vi "单参数加标流程.vi"(10 "流程类型":T4, 11 "Slave ID":T6=enum."氨氮") -> ()   [LabVIEW 2016, in "质控单元V4.lvlib"]
panel:
  in  "平行样测试数据":T1={"时间"=timestamp(0 s since 1904-01-01), "参数"="", "数据类型"="N", "第一次水样浓度值"=0.0, "第二次水样测试时间"=timestamp(0 s since 1904-01-01), "第二次水样浓度值"=0.0}
  in  "集成干预测试数据":T2={"时间"=timestamp(0 s since 1904-01-01), "参数"="", "数据类型"="N", "集成干预测试浓度值"=0.0, "集成干预前测试时间"=timestamp(0 s since 1904-01-01), "集成干预前测试浓度值"=0.0}
  out "平行样启动时间":timestamp
  out "加标模块润洗流程控制":T3=enum."启动水样润洗流程"
  in  "获取加标回收测试数据计数":u16
  in  "获取水样测试数据计数":u16
  in  "写入加标体积重试次数":u16
  in  "加标模块加标润洗启动计数":u16
  out "加标回收启动时间":timestamp
  out "水样测试启动时间":timestamp
  out "Next State":string
  in  "仪器加标回收启动计数":u16
  in  "仪器水样测试启动计数":u16
  in  "加标模块排液启动计数":u16
  in  "加标模块加标启动计数":u16
  in  "加标模块进样启动计数":u16
  in  "加标模块水样润洗启动计数":u16
  in  "采配水启动次数计数":u16
  in  "加标回收测试时间":timestamp
  in  "水样测试时间":timestamp
  in  "质控数据":T5
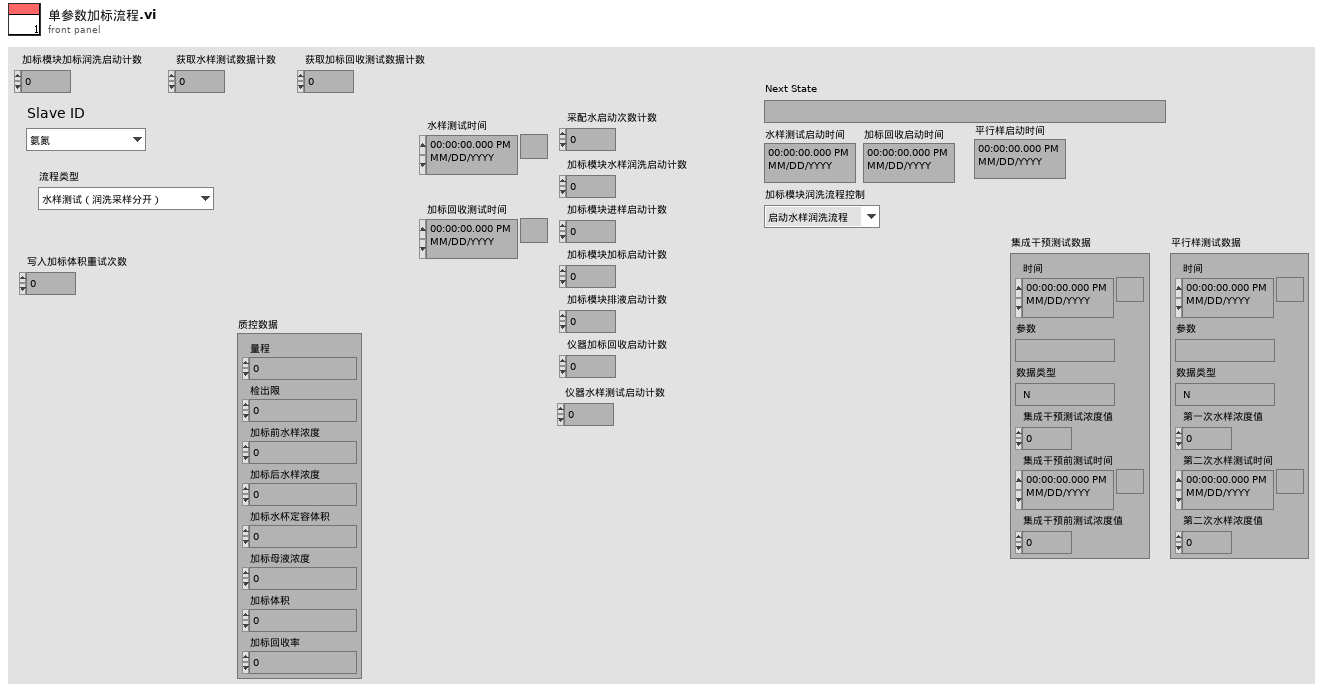
[diagram p1: front panel]
types:
  T1 = typedef "平行样测试数据字段定义.ctl" = cluster{"时间":timestamp, "参数":string, "数据类型":string, "第一次水样浓度值":dbl, "第二次水样测试时间":timestamp, "第二次水样浓度值":dbl}
  T2 = typedef "集成干预字段定义.ctl" = cluster{"时间":timestamp, "参数":string, "数据类型":string, "集成干预测试浓度值":dbl, "集成干预前测试时间":timestamp, "集成干预前测试浓度值":dbl}
  T3 = typedef "质控单元V4.lvlib/质控流程控制.ctl" = enum16{"待机", "启动进样流程", "启动加标流程", "启动排液流程", "启动水样润洗流程", "启动加标润洗流程", "停止流程"}
  T4 = typedef "质控单元V4.lvlib/测试子流程.ctl" = enum16{"水样测试（润洗采样分开）", "水样测试（润洗采样合并）", "水样测试（不启动采配水）", "加标回收（润洗采样分开）", "加标回收（润洗采样合并）", "加标回收（不启动采配水）", "集成干预测试", "平行样测试", "平行样测试（不启动采配水）", "水样测试（不含采样杯）", "平行样测试（不含采样杯）", "集成干预测试（不含采样杯）"}
  T5 = cluster{"量程":dbl, "检出限":dbl, "加标前水样浓度":dbl, "加标后水样浓度":dbl, "加标水杯定容体积":dbl, "加标母液浓度":dbl, "加标体积":dbl, "加标回收率":dbl}
  T6 = typedef "质控单元V4.lvlib/质控slave id.ctl" = enum16{"null", "氨氮", "总磷", "总氮", "CODMn", "CODCr"}
  T7 = cluster{"氨氮":bool, "总磷":bool, "总氮":bool, "CODMn":bool, "CODCr":bool}
  T8 = cluster{"时间":timestamp, "参数":string, "数据类型":string, "加标回收率":sgl, "加标前水样测试时间":timestamp, "加标前水样浓度值":sgl, "加标后水样浓度值":sgl, "加标母液浓度值":sgl, "加标体积":sgl, "加标水杯定容体积":sgl}
  T9 = enum16{"待机", "水样测试（全流程）", "停止", "加标回收", "水样测试（简易流程）"}
  T10 = enum16{"待机", "润洗", "采样", "沉淀", "配水", "反冲洗", "储水", "结束"}
  T11 = typedef "质控单元V4.lvlib/采配水通用流程.ctl" = enum16{"待机", "润洗", "采样", "沉淀", "配水", "反冲洗", "结束"}
  T12 = typedef "质控单元V4.lvlib/质控组合命令区.ctl" = enum16{"停止", "进水样", "排废液", "进空气（搅拌）", "定量（反转定量）"}
  T13 = enum16{"待机", "润洗", "进样", "定量", "加标", "等待取样", "排液", "异常停机"}
  T14 = enum16{"空闲", "水样测试", "标样核查", "零点核查", "跨度核查", "空白测试", "平行样测试", "加标回收", "空白校准", "标样校准", "初始化（清洗）"}
  T15 = cluster{"时间":timestamp, "参数":string, "数据类型":string, "第一次水样浓度值":dbl, "第二次水样测试时间":timestamp, "第二次水样浓度值":dbl}
  T16 = cluster{"水样数据时间":timestamp, "水样实测值":sgl, "水样数据标识":string}
  T17 = cluster{"加标回收数据时间":timestamp, "加标回收实测值":sgl, "加标回收数据标识":string}
  T18 = typedef "质控单元V4.lvlib/质控仪器状态.ctl" = cluster{"运行状态":enum16{"待机", "润洗", "进样", "定量", "加标", "等待取样", "排液", "异常停机"}, "液位状态":enum16{"无感应", "有感应"}, "告警状态":enum16{"无告警", "液位故障告警", "注射泵异常"}, "当前步骤数":u16, "当前步骤剩余时间":u16, "当前步骤具体操作":enum16{"加标", "进样", "排液", "搅拌", "定量"}, "当前流程":enum16{"待机", "进样流程", "加标流程", "排液流程", "水样润洗流程", "加标润洗流程"}}
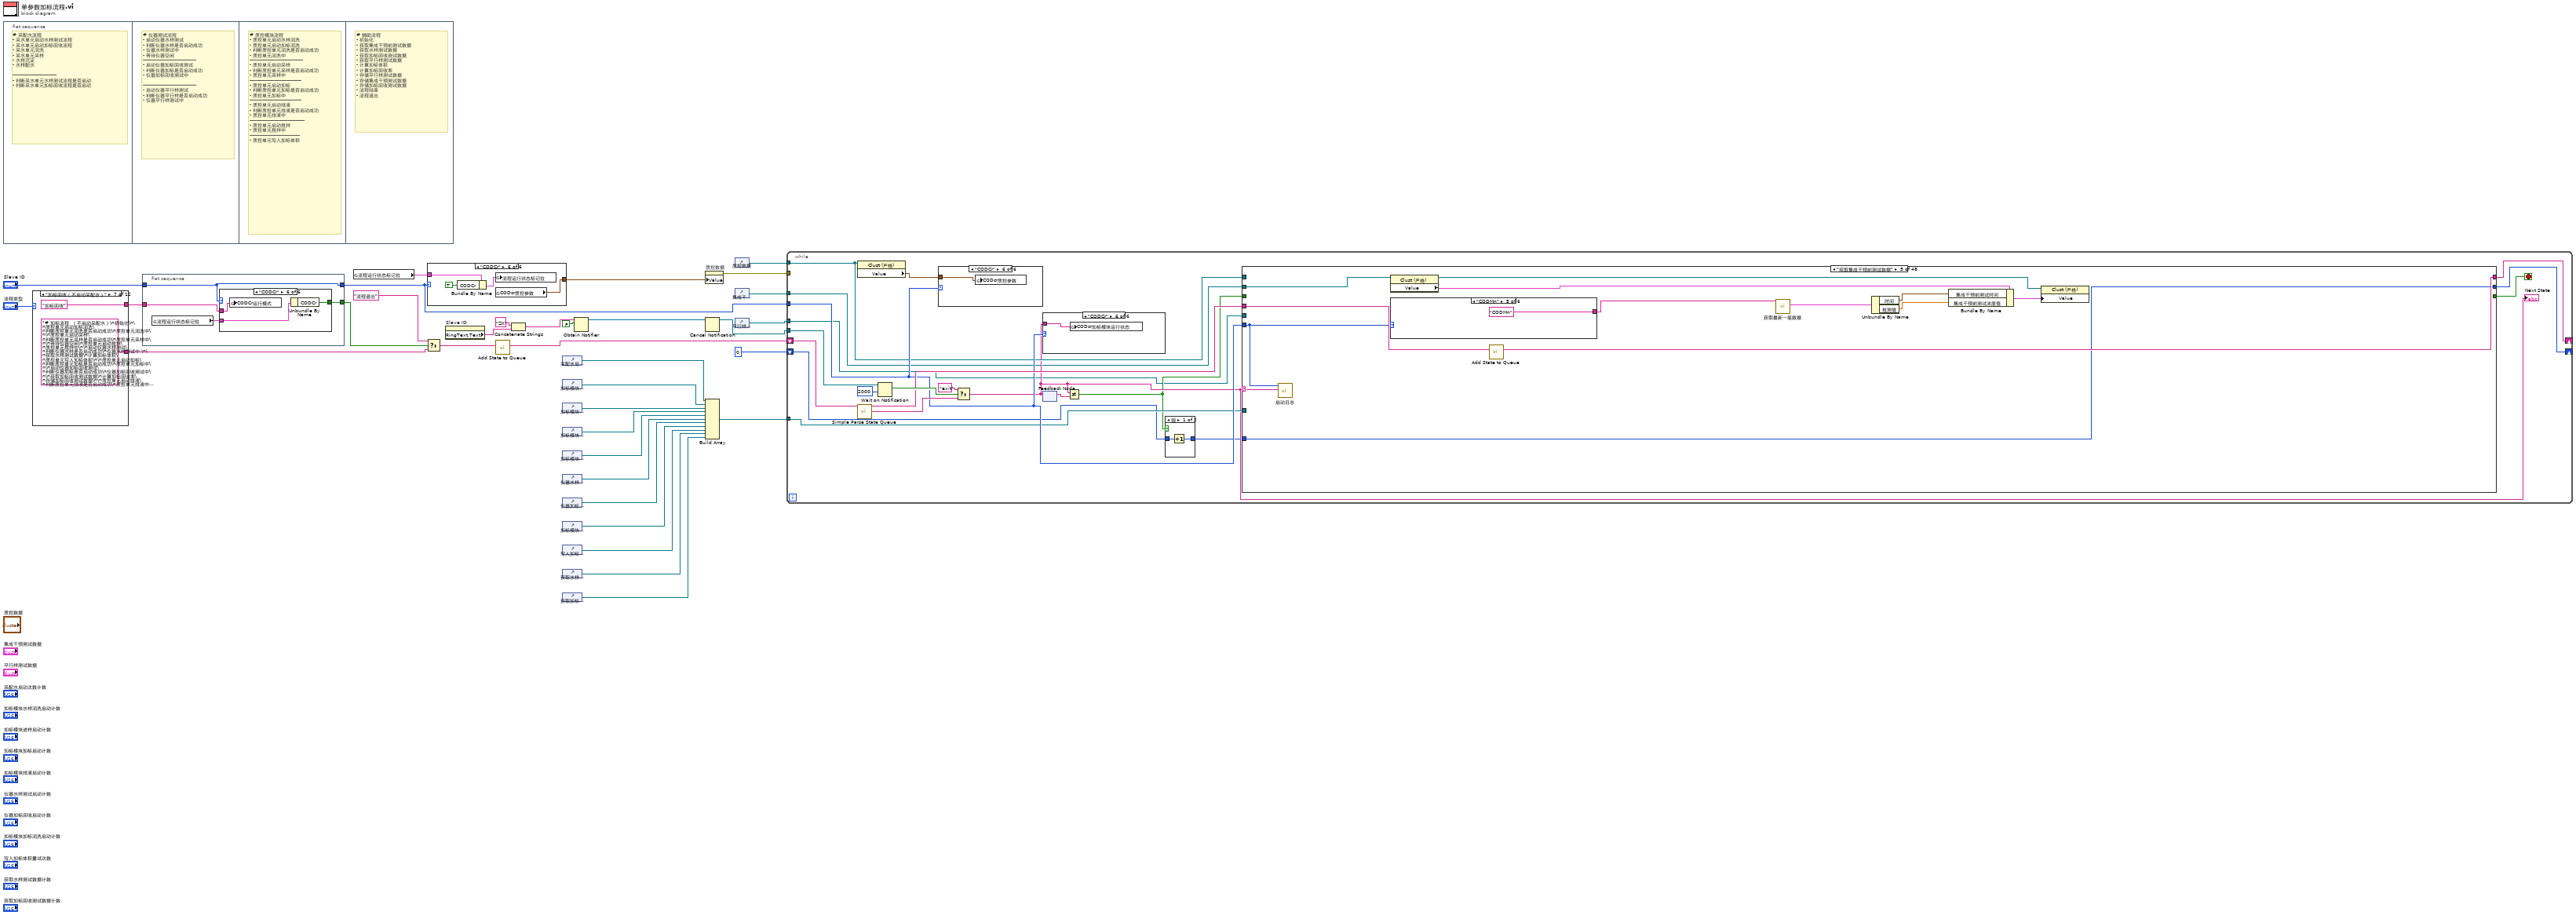
[diagram p0: block diagram]
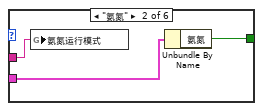
[diagram p3: hidden frame]
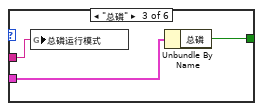
[diagram p4: hidden frame]
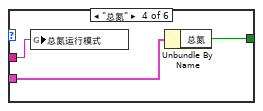
[diagram p5: hidden frame]
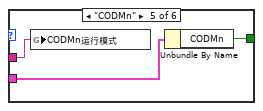
[diagram p6: hidden frame]
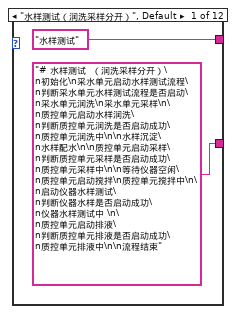
[diagram p7: hidden frame]
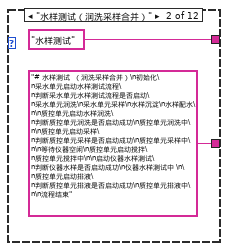
[diagram p8: hidden frame]
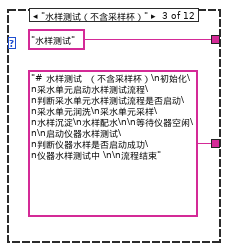
[diagram p9: hidden frame]
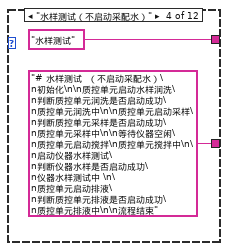
[diagram p10: hidden frame]
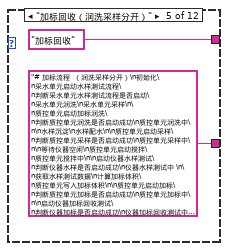
[diagram p11: hidden frame]
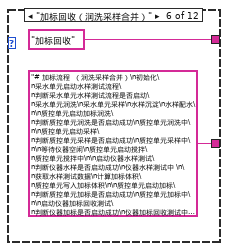
[diagram p12: hidden frame]
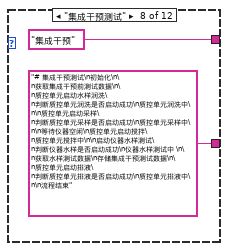
[diagram p13: hidden frame]
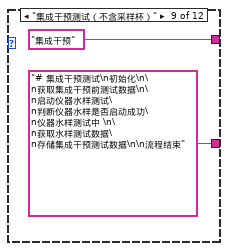
[diagram p14: hidden frame]
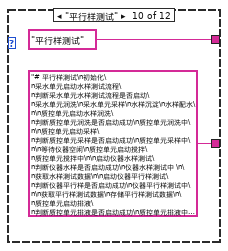
[diagram p15: hidden frame]
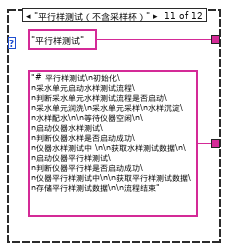
[diagram p16: hidden frame]
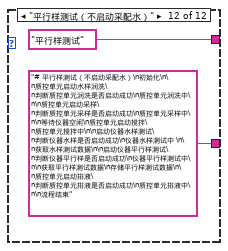
[diagram p17: hidden frame]
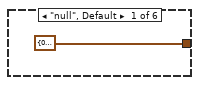
[diagram p18: hidden frame]
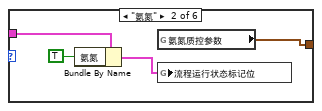
[diagram p19: hidden frame]
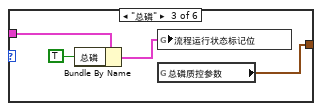
[diagram p20: hidden frame]
diagram:
  n1 = flat-sequence {
    frame #0 {
      # "# 采配水流程\n- 采水单元启动水样测试流程\n- 采水单元启动加标回收流程\n- 采水单元润洗\n- 采水单元采样 \n- 水样沉淀\n- 水样配水\n\n----------------------------\n- 判断采水单元水样测试流程是否启动\n- 判断采水单元加标回收流程是否启动"
    }
    frame #1 {
      # "# 仪器测试流程\n- 启动仪器水样测试\n- 判断仪器水样是否启动成功\n- 仪器水样测试中\n- 等待仪器空闲\n----------------------------------\n- 启动仪器加标回收测试\n- 判断仪器加标是否启动成功\n- 仪器加标回收测试中\n\n----------------------------------\n- 启动仪器平行样测试\n- 判断仪器平行样是否启动成功\n- 仪器平行样测试中"
    }
    frame #2 {
      # "# 质控模块流程\n- 质控单元启动水样润洗\n- 质控单元启动加标润洗\n- 判断质控单元润洗是否启动成功\n- 质控单元润洗中\n----------------------------------\n- 质控单元启动采样\n- 判断质控单元采样是否启动成功\n- 质控单元采样中\n---------------------------------\n- 质控单元启动加标\n- 判断质控单元加标是否启动成功\n- 质控单元加标中\n---------------------------------\n- 质控单元启动排液\n- 判断质控单元排液是否启动成功\n- 质控单元排液中\n-----------------------------------\n- 质控单元启动搅拌\n- 质控单元搅拌中\n--------------------------------\n- 质控单元写入加标体积"
    }
    frame #3 {
      # "# 辅助流程\n- 初始化\n- 获取集成干预前测试数据\n- 获取水样测试数据\n- 获取加标回收测试数据\n- 获取平行样测试数据\n- 计算加标体积\n- 计算加标回收率\n- 存储平行样测试数据\n- 存储集成干预测试数据\n- 存储加标回收测试数据 \n- 流程结束\n- 流程退出"
    }
  }
  n2 = case shown="\"加标回收（不启动采配水）\"" "流程类型" {
    tunnel: ["# 水样测试  （润洗采样分开）\n初始化\n采水单元启动水样测试流程\n判断采水单元水样测试流程是否启动\n采水单元润洗\n采水单元采样\n\n质控单元启动水样润洗\n判断质控单元润洗是否启动成功\n质控单元润洗中\n\n水样沉淀\n水样配水\n\n质控单元启动采样\n判断质控单元采样是否启动成功\n质控单元采样中\n\n等待仪器空闲\n质控单元启动搅拌\n质控单元搅拌中\n\n启动仪器水样测试\n判断仪器水样是否启动成功\n仪器水样测试中 \n\n质控单元启动排液\n判断质控单元排液是否启动成功\n质控单元排液中\n\n流程结束" ("State(s) In (\"\")") "# 水样测试  （润洗采样合并）\n初始化\n采水单元启动水样测试流程\n判断采水单元水样测试流程是否启动\n采水单元润洗\n采水单元采样\n水样沉淀\n水样配水\n\n质控单元启动水样润洗\n判断质控单元润洗是否启动成功\n质控单元润洗中\n\n质控单元启动采样\n判断质控单元采样是否启动成功\n质控单元采样中\n\n等待仪器空闲\n质控单元启动搅拌\n质控单元搅拌中\n\n启动仪器水样测试\n判断仪器水样是否启动成功\n仪器水样测试中 \n\n质控单元启动排液\n判断质控单元排液是否启动成功\n质控单元排液中\n\n流程结束" ("State(s) In (\"\")") "# 水样测试  （不含采样杯）\n初始化\n采水单元启动水样测试流程\n判断采水单元水样测试流程是否启动\n采水单元润洗\n采水单元采样\n水样沉淀\n水样配水\n\n等待仪器空闲\n\n启动仪器水样测试\n判断仪器水样是否启动成功\n仪器水样测试中 \n\n流程结束" ("State(s) In (\"\")") "# 水样测试  （不启动采配水）\n初始化\n\n质控单元启动水样润洗\n判断质控单元润洗是否启动成功\n质控单元润洗中\n\n质控单元启动采样\n判断质控单元采样是否启动成功\n质控单元采样中\n\n等待仪器空闲\n质控单元启动搅拌\n质控单元搅拌中\n\n启动仪器水样测试\n判断仪器水样是否启动成功\n仪器水样测试中 \n\n质控单元启动排液\n判断质控单元排液是否启动成功\n质控单元排液中\n\n流程结束" ("State(s) In (\"\")") "# 加标流程  （润洗采样分开）\n初始化\n采水单元启动水样测试流程\n判断采水单元水样测试流程是否启动\n采水单元润洗\n采水单元采样\n\n质控单元启动加标润洗\n判断质控单元润洗是否启动成功\n质控单元润洗中\n\n水样沉淀\n水样配水\n\n质控单元启动采样\n判断质控单元采样是否启动成功\n质控单元采样中\n\n等待仪器空闲\n质控单元启动搅拌\n质控单元搅拌中\n\n启动仪器水样测试\n判断仪器水样是否启动成功\n仪器水样测试中 \n\n获取水样测试数据\n计算加标体积\n质控单元写入加标体积\n\n质控单元启动加标\n判断质控单元加标是否启动成功\n质控单元加标中\n\n启动仪器加标回收测试\n判断仪器加标是否启动成功\n仪器加标回收测试中\n\n获取加标回收测试数据\n计算加标回收率\n存储加标回收测试数据\n\n质控单元启动排液\n判断质控单元排液是否启动成功\n质控单元排液中\n\n流程结束" ("State(s) In (\"\")") "# 加标流程  （润洗采样合并）\n初始化\n采水单元启动水样测试流程\n判断采水单元水样测试流程是否启动\n采水单元润洗\n采水单元采样\n水样沉淀\n水样配水\n\n质控单元启动加标润洗\n判断质控单元润洗是否启动成功\n质控单元润洗中\n\n质控单元启动采样\n判断质控单元采样是否启动成功\n质控单元采样中\n\n等待仪器空闲\n质控单元启动搅拌\n质控单元搅拌中\n\n启动仪器水样测试\n判断仪器水样是否启动成功\n仪器水样测试中 \n\n获取水样测试数据\n计算加标体积\n质控单元写入加标体积\n\n质控单元启动加标\n判断质控单元加标是否启动成功\n质控单元加标中\n\n启动仪器加标回收测试\n判断仪器加标是否启动成功\n仪器加标回收测试中\n\n获取加标回收测试数据\n计算加标回收率\n存储加标回收测试数据\n\n质控单元启动排液\n判断质控单元排液是否启动成功\n质控单元排液中\n\n流程结束" ("State(s) In (\"\")") "# 加标流程  （不启动采配水）\n初始化\n\n质控单元启动加标润洗\n判断质控单元润洗是否启动成功\n质控单元润洗中\n\n质控单元启动采样\n判断质控单元采样是否启动成功\n质控单元采样中\n\n等待仪器空闲\n质控单元启动搅拌\n质控单元搅拌中\n\n启动仪器水样测试\n判断仪器水样是否启动成功\n仪器水样测试中 \n\n获取水样测试数据\n计算加标体积\n质控单元写入加标体积\n\n质控单元启动加标\n判断质控单元加标是否启动成功\n质控单元加标中\n\n启动仪器加标回收测试\n判断仪器加标是否启动成功\n仪器加标回收测试中\n\n获取加标回收测试数据\n计算加标回收率\n存储加标回收测试数据\n\n质控单元启动排液\n判断质控单元排液是否启动成功\n质控单元排液中\n\n流程结束" ("State(s) In (\"\")") "# 集成干预测试\n初始化\n\n获取集成干预前测试数据\n\n质控单元启动水样润洗\n判断质控单元润洗是否启动成功\n质控单元润洗中\n\n质控单元启动采样\n判断质控单元采样是否启动成功\n质控单元采样中\n\n等待仪器空闲\n质控单元启动搅拌\n质控单元搅拌中\n\n启动仪器水样测试\n判断仪器水样是否启动成功\n仪器水样测试中 \n\n获取水样测试数据\n存储集成干预测试数据\n\n质控单元启动排液\n判断质控单元排液是否启动成功\n质控单元排液中\n\n流程结束" ("State(s) In (\"\")") "# 集成干预测试\n初始化\n\n获取集成干预前测试数据\n\n启动仪器水样测试\n判断仪器水样是否启动成功\n仪器水样测试中 \n\n获取水样测试数据\n存储集成干预测试数据\n\n流程结束" ("State(s) In (\"\")") "# 平行样测试\n初始化\n采水单元启动水样测试流程\n判断采水单元水样测试流程是否启动\n采水单元润洗\n采水单元采样\n水样沉淀\n水样配水\n\n质控单元启动水样润洗\n判断质控单元润洗是否启动成功\n质控单元润洗中\n\n质控单元启动采样\n判断质控单元采样是否启动成功\n质控单元采样中\n\n等待仪器空闲\n质控单元启动搅拌\n质控单元搅拌中\n\n启动仪器水样测试\n判断仪器水样是否启动成功\n仪器水样测试中 \n\n获取水样测试数据\n\n启动仪器平行样测试\n判断仪器平行样是否启动成功\n仪器平行样测试中\n\n获取平行样测试数据\n存储平行样测试数据\n\n质控单元启动排液\n判断质控单元排液是否启动成功\n质控单元排液中\n\n流程结束" ("State(s) In (\"\")") "# 平行样测试\n初始化\n采水单元启动水样测试流程\n判断采水单元水样测试流程是否启动\n采水单元润洗\n采水单元采样\n水样沉淀\n水样配水\n\n等待仪器空闲\n\n启动仪器水样测试\n判断仪器水样是否启动成功\n仪器水样测试中 \n\n获取水样测试数据\n\n启动仪器平行样测试\n判断仪器平行样是否启动成功\n仪器平行样测试中\n\n获取平行样测试数据\n存储平行样测试数据\n\n流程结束" ("State(s) In (\"\")") "# 平行样测试（不启动采配水）\n初始化\n\n质控单元启动水样润洗\n判断质控单元润洗是否启动成功\n质控单元润洗中\n\n质控单元启动采样\n判断质控单元采样是否启动成功\n质控单元采样中\n\n等待仪器空闲\n质控单元启动搅拌\n质控单元搅拌中\n\n启动仪器水样测试\n判断仪器水样是否启动成功\n仪器水样测试中 \n\n获取水样测试数据\n\n启动仪器平行样测试\n判断仪器平行样是否启动成功\n仪器平行样测试中\n\n获取平行样测试数据\n存储平行样测试数据\n\n质控单元启动排液\n判断质控单元排液是否启动成功\n质控单元排液中\n\n流程结束" ("State(s) In (\"\")")] -> w12
    tunnel: ["水样测试" "水样测试" "水样测试" "水样测试" "加标回收" "加标回收" "加标回收" "集成干预" "集成干预" "平行样测试" "平行样测试" "平行样测试"] -> w6
    frame "水样测试（润洗采样分开）", Default {
    }
    frame "水样测试（润洗采样合并）" {
    }
    frame "水样测试（不含采样杯）" {
    }
    frame "水样测试（不启动采配水）" {
    }
    frame "加标回收（润洗采样分开）" {
    }
    frame "加标回收（润洗采样合并）" {
    }
    frame "加标回收（不启动采配水）" {
    }
    frame "集成干预测试" {
    }
    frame "集成干预测试（不含采样杯）" {
    }
    frame "平行样测试" {
    }
    frame "平行样测试（不含采样杯）" {
    }
    frame "平行样测试（不启动采配水）" {
    }
  }
  n3 = flat-sequence {
    tunnel: [w60] -> w15
    tunnel: [w61] -> w14
    tunnel: "Slave ID" -> [w60]
    tunnel: w6 -> [w59]
    frame #0 {
      n4 = global read "ZK非断电保存全局变量.vi" "流程运行状态标记位"() -> (w62:T7)
      n5 = case shown="\"CODCr\"" w60 {
        tunnel: w62 -> [_ w65 w68 w71 w74 w77]
        tunnel: [_ w64 w67 w70 w73 w76] -> w61
        tunnel: w59 -> [_ w63 w66 w69 w72 w75]
        frame "null", Default {
        }
        frame "氨氮" {
          n6 = global write "ZK非断电保存全局变量.vi" "氨氮运行模式"(w63) -> ()
          n7 = Unbundle By Name(w65) -> ("氨氮"=w64:bool)
        }
        frame "总磷" {
          n8 = global write "ZK非断电保存全局变量.vi" "总磷运行模式"(w66) -> ()
          n9 = Unbundle By Name(w68) -> ("总磷"=w67:bool)
        }
        frame "总氮" {
          n10 = global write "ZK非断电保存全局变量.vi" "总氮运行模式"(w69) -> ()
          n11 = Unbundle By Name(w71) -> ("总氮"=w70:bool)
        }
        frame "CODMn" {
          n12 = global write "ZK非断电保存全局变量.vi" "CODMn运行模式"(w72) -> ()
          n13 = Unbundle By Name(w74) -> ("CODMn"=w73:bool)
        }
        frame "CODCr" {
          n14 = global write "ZK非断电保存全局变量.vi" "CODCr运行模式"(w75) -> ()
          n15 = Unbundle By Name(w77) -> ("CODCr"=w76:bool)
        }
      }
    }
  }
  n16 = global read "ZK非断电保存全局变量.vi" "流程运行状态标记位"() -> (w17:T7)
  n17 = Select(t="流程退出", s=w14, f=w12) -> (s? t:f=w11:string)
  n18 = case shown="\"CODCr\"" w15 {
    tunnel: [T5 {"量程"=0.0, "检出限"=0.0, "加标前水样浓度"=0.0, "加标后水样浓度"=0.0, "加标水杯定容体积"=0.0, "加标母液浓度"=0.0, "加标体积"=0.0, "加标回收率"=0.0} ("CODcr质控参数") w82 w86 w90 w94 w98] -> w26
    tunnel: w17 -> [_ w81 w83 w87 w91 w95]
    frame "null", Default {
    }
    frame "氨氮" {
      n19 = Bundle By Name(cluster=w81, "氨氮"=TRUE) -> (w80:T7)
      n20 = global read "ZK断电保存全局变量.vi" "氨氮质控参数"() -> (w82:T5)
      n21 = global write "ZK非断电保存全局变量.vi" "流程运行状态标记位"(w80) -> ()
    }
    frame "总磷" {
      n22 = Bundle By Name(cluster=w83, "总磷"=TRUE ("氨氮")) -> (w85:T7)
      n23 = global write "ZK非断电保存全局变量.vi" "流程运行状态标记位"(w85) -> ()
      n24 = global read "ZK断电保存全局变量.vi" "总磷质控参数"() -> (w86:T5)
    }
    frame "总氮" {
      n25 = Bundle By Name(cluster=w87, "总氮"=TRUE ("氨氮")) -> (w89:T7)
      n26 = global write "ZK非断电保存全局变量.vi" "流程运行状态标记位"(w89) -> ()
      n27 = global read "ZK断电保存全局变量.vi" "总氮质控参数"() -> (w90:T5)
    }
    frame "CODMn" {
      n28 = Bundle By Name(cluster=w91, "CODMn"=TRUE ("氨氮")) -> (w93:T7)
      n29 = global write "ZK非断电保存全局变量.vi" "流程运行状态标记位"(w93) -> ()
      n30 = global read "ZK断电保存全局变量.vi" "CODMn质控参数"() -> (w94:T5)
    }
    frame "CODCr" {
      n31 = Bundle By Name(cluster=w95, "CODCr"=TRUE ("氨氮")) -> (w97:T7)
      n32 = global write "ZK非断电保存全局变量.vi" "流程运行状态标记位"(w97) -> ()
      n33 = global read "ZK断电保存全局变量.vi" "CODcr质控参数"() -> (w98:T5)
    }
  }
  n34 = property on="Slave ID" class="Enum (严格)"() -> ("RingText.Text"=w34:string)  [unwired: 2 in, 2 out]
  n35 = call "Add State to Queue.vi"("State(s) In (\"\")"=w11) -> ("States Out"=w28:string)  [unwired: 14 in]
  n36 = Concatenate Strings("ZK" ("字符串"), w34) -> (w32:string)
  n37 = control-ref of="采配水启动次数计数"() -> (w24:refnum<vi>)
  n38 = control-ref of="加标模块水样润洗启动计数"() -> (w23:refnum<vi>)
  n39 = control-ref of="加标模块进样启动计数"() -> (w22:refnum<vi>)
  n40 = control-ref of="加标模块加标启动计数"() -> (w21:refnum<vi>)
  n41 = control-ref of="加标模块排液启动计数"() -> (w20:refnum<vi>)
  n42 = control-ref of="仪器水样测试启动计数"() -> (w4:refnum<vi>)
  n43 = control-ref of="仪器加标回收启动计数"() -> (w5:refnum<vi>)
  n44 = control-ref of="加标模块加标润洗启动计数"() -> (w16:refnum<vi>)
  n45 = control-ref of="写入加标体积重试次数"() -> (w10:refnum<vi>)
  n46 = control-ref of="获取水样测试数据计数"() -> (w9:refnum<vi>)
  n47 = control-ref of="获取加标回收测试数据计数"() -> (w8:refnum<vi>)
  n48 = Obtain Notifier(name (unnamed)=w32, notification data type=FALSE) -> (notifier out=w30:refnum<notifier>)  [unwired: 2 in, 2 out]
  n49 = property on="质控数据" class="Clust (严格)"("Value"=w26) -> (error out=w27:errorcluster)  [unwired: 2 in, 1 out]
  n50 = Cancel Notification(0:w30) -> (8:w29:refnum<notifier>)  [unwired: 1 in, 2 out]
  n51 = Build Array(w24, w23, w22, w21, w20, w4, w5, w16, w10, w9, w8) -> (w19:refnum<vi>[])
  n52 = control-ref of="质控数据"() -> (w25:refnum<vi>)
  n53 = control-ref of="集成干预测试数据"() -> (w2:refnum<vi>)
  n54 = control-ref of="平行样测试数据"() -> (w1:refnum<vi>)
  n55 = while {
    tunnel: w29 -> [w118]
    tunnel: w15 -> [w110]
    shift-right: [w112] -> _
    shift-left: w28 -> [w119]
    tunnel: w27 -> [_]
    tunnel: w25 -> [w109]
    tunnel: w19 -> [w107]
    shift-right: [w102] -> _
    shift-left: 0 -> [w104]
    tunnel: w2 -> [w99]
    tunnel: w1 -> [w100]
    stop <- w111 stop-if-true
    n56 = property class="Clust (严格)"(reference=w109) -> ("Value"=w108:T5)  [unwired: 1 in, 2 out]
    n57 = call "Simple Parse State Queue.vi"("State Queue"=w119) -> ("Remain States"=w113:string, "Next State"=w115:string)  [unwired: 13 in]
    n58 = Wait on Notification(notifier=w118, timeout in ms (-1)=2000 ("超时毫秒(-1)")) -> (notification=w116:bool)  [unwired: 2 in, 3 out]
    n59 = case shown="\"CODCr\"" w110 {
      tunnel: w108 -> [_ w122 w123 w124 w125 w126]
      frame "null", Default {
      }
      frame "氨氮" {
        n60 = global write "ZK断电保存全局变量.vi" "氨氮质控参数"(w122) -> ()
      }
      frame "总磷" {
        n61 = global write "ZK断电保存全局变量.vi" "总磷质控参数"(w123) -> ()
      }
      frame "总氮" {
        n62 = global write "ZK断电保存全局变量.vi" "总氮质控参数"(w124) -> ()
      }
      frame "CODMn" {
        n63 = global write "ZK断电保存全局变量.vi" "CODMn质控参数"(w125) -> ()
      }
      frame "CODCr" {
        n64 = global write "ZK断电保存全局变量.vi" "CODcr质控参数"(w126) -> ()
      }
    }
    n65 = Select(t="exit" ("State(s) In (\"\")"), s=w116, f=w115) -> (s? t:f=w105:string)
    "Next State" <- w105
    n66 = case shown="\"CODCr\"" w110 {
      tunnel: w105 -> [_ w127 w128 w129 w130 w131]
      frame "null", Default {
      }
      frame "氨氮" {
        n67 = global write "ZK非断电保存全局变量.vi" "氨氮加标模块运行状态"(w127) -> ()
      }
      frame "总磷" {
        n68 = global write "ZK非断电保存全局变量.vi" "总磷加标模块运行状态"(w128) -> ()
      }
      frame "总氮" {
        n69 = global write "ZK非断电保存全局变量.vi" "总氮加标模块运行状态"(w129) -> ()
      }
      frame "CODMn" {
        n70 = global write "ZK非断电保存全局变量.vi" "CODMn加标模块运行状态"(w130) -> ()
      }
      frame "CODCr" {
        n71 = global write "ZK非断电保存全局变量.vi" "CODcr加标模块运行状态"(w131) -> ()
      }
    }
    n72 = feedback-in #1(w105) -> ()
    n73 = feedback #1() -> (w106:string)  [unwired: 1 in]
    n74 = Not Equal?(x=w105, y=w106) -> (x != y?=w101:bool)
    n75 = case shown="假" w101 {
      tunnel: w104 -> [w121 _]
      tunnel: [w120 _] -> w103
      frame False {
        n76 = Increment(x=w121) -> (x+1=w120:i32)
      }
      frame True {
      }
    }
    n77 = case shown="\"获取集成干预前测试数据\"" w105 {
      selector: w105 -> [_ _ w143 w168 w225 w235 w289 w340 w350 w361 w388 w405 w417 w447 _ w457 w468 w480 w501 w523 w544 w565 w587 _ w604 w617 w628 w646 w666 w678 w693 w696 w739 w778 w817 w866 w898 w930 _ w945 w962 w980 w998 w1017 w1053 w1091 w1131 w1171]
      tunnel: w113 -> [w134 w137 w152 w190 w227 w261 w313 w348 w357 w375 w391 w407 w423 w451 w454 w465 w476 w495 w502 w535 w553 w573 w595 w602 w614 w626 w638 w653 w676 w688 w695 w720 w761 w800 w839 w875 w908 w933 w941 w954 w966 w989 w1007 w1019 w1070 w1109 w1148 w1177]
      tunnel: [w133 w136 w151 w189 w226 w260 w312 w347 w356 w374 w390 w406 w422 w450 w453 w464 w475 w494 w516 w534 w552 w572 w594 w601 w613 w625 w637 w652 w675 w687 w694 w719 w760 w799 w838 w874 w907 w932 w940 w953 w965 w988 w1006 w1018 w1069 w1108 w1147 w1176] -> w112
      tunnel: [_ _ _ _ _ _ _ _ _ _ _ _ TRUE TRUE _ _ _ _ _ _ _ _ _ _ _ _ _ _ _ _ _ _ _ _ _ _ _ _ _ _ _ _ _ _ _ _ _ _] -> w111
      tunnel: w110 -> [_ _ w142 w177 w219 w246 w300 w339 w351 w362 w389 w400 w418 w448 _ w458 w469 w479 w500 w522 w542 w562 w585 _ w605 w618 w629 w640 w667 w679 w690 w705 w746 w785 w824 w860 w896 w925 _ w946 w963 w981 w999 w1015 w1056 w1095 w1134 w1170]
      tunnel: w109 -> [_ _ w148 w188 _ w259 _ w346 w355 w373 _ _ _ _ _ _ _ _ _ _ _ _ _ _ _ _ _ w651 _ _ _ _ _ _ _ _ _ _ _ _ _ _ _ _ _ _ _ _]
      tunnel: w107 -> [_ _ w139 w174 _ w237 w291 _ _ _ _ _ _ _ _ w463 w474 w484 w506 _ _ _ _ _ w607 w620 w631 w645 w670 w682 _ w710 w751 w790 w829 _ _ _ _ w949 _ w984 w1002 _ w1061 w1101 w1140 _]
      tunnel: w103 -> [w132 w135 w138 w165 w224 w234 w288 w338 w349 w358 w387 w404 w414 w444 w452 w456 w467 w477 w498 w520 w541 w560 w584 w600 w603 w615 w627 w639 w665 w677 w689 w703 w744 w784 w822 w858 w894 w928 w939 w943 w964 w978 w996 w1014 w1055 w1094 w1133 w1167]
      tunnel: [w132 w135 w138 w165 w224 w234 w288 w338 w349 w358 w387 w404 w414 w444 w452 w456 w467 w477 w498 w520 w541 w560 w584 w600 w603 w615 w627 w639 w665 w677 w689 w703 w744 w784 w822 w858 w894 w928 w939 w943 w964 w978 w996 w1014 w1055 w1094 w1133 w1167] -> w102
      tunnel: w101 -> [_ _ _ _ _ _ _ _ _ _ _ _ _ _ _ _ _ _ _ w519 w540 w559 w583 _ _ _ _ _ _ _ _ w700 w745 w783 w823 w859 w895 w924 _ _ w960 _ _ _ w1052 w1092 w1130 w1168]
      tunnel: w100 -> [_ _ _ w163 _ _ w287 _ _ _ w386 _ _ _ _ _ _ _ _ _ _ _ _ _ _ _ _ _ _ _ _ _ _ _ _ _ _ _ _ _ _ _ _ _ _ _ _ _]
      tunnel: w99 -> [_ _ _ w157 w220 _ _ _ _ _ _ w403 _ _ _ _ _ _ _ _ _ _ _ _ _ _ _ _ _ _ _ _ _ _ _ _ _ _ _ _ _ _ _ _ _ _ _ _]
      frame Default {
        n78 = call "Add State to Queue.vi"("State(s) In (\"\")"=w134) -> ("States Out"=w133:string)  [unwired: 14 in]
      }
      frame "-------------------# 辅助流程 #-------------------" {
        n79 = call "Add State to Queue.vi"("State(s) In (\"\")"=w137) -> ("States Out"=w136:string)  [unwired: 14 in]
      }
      frame "初始化" {
        w144 = 0.0 ("加标前水样浓度")
        n80 = call "ZK报警清除.vi"("Slave ID"=w142) -> ()  [unwired: 10 in, 1 out]
        n81 = local write "加标回收测试时间"(timestamp(0 s since 1904-01-01) ("加标回收测试时间")) -> ()
        n82 = for {
          tunnel: w139 -> [w154] mode=indexing
          n83 = property class="DigNum (严格)"(reference=w154, "Value"=u16 0 ("值")) -> ()  [unwired: 1 in, 2 out]
        }
        n84 = property class="Clust (严格)"(reference=w148) -> (reference out=w147:refnum<vi>, "Value"=w146:T5)  [unwired: 1 in, 1 out]
        n85 = Concatenate Strings("----->>" ("字符串"), w143) -> (w141:string)
        n86 = local write "水样测试时间"(timestamp(0 s since 1904-01-01) ("水样测试时间")) -> ()
        n87 = call "启动日志.vi"("日志信息"=w141, "Slave ID"=w142) -> ()  [unwired: 9 in, 1 out]
        n88 = Bundle By Name(cluster=w146, "加标前水样浓度"=w144, "加标后水样浓度"=w144, "加标体积"=w144, "加标回收率"=w144) -> (w145:T5)
        n89 = property class="Clust (严格)"(reference=w147, "Value"=w145) -> ()  [unwired: 1 in, 2 out]
        n90 = call "Add State to Queue.vi"("State(s) In (\"\")"=w152) -> ("States Out"=w151:string)  [unwired: 14 in]
      }
      frame "获取水样测试数据" {
        n91 = call "启动日志.vi"("日志信息"=w168, "Slave ID"=w177) -> ()  [unwired: 9 in, 1 out]
        n92 = property class="Clust (严格)"(reference=w163) -> (reference out=w164:refnum<vi>, "Value"=w162:T15)  [unwired: 1 in, 1 out]
        n93 = case shown="\"CODCr\"" w177 {
          tunnel: [sgl 0.0 ("水样实测值") w198 w202 w206 w210 w214] -> w155
          tunnel: [timestamp(0 s since 1904-01-01) ("水样数据时间") w197 w201 w205 w209 w213] -> w156
          frame "null", Default {
          }
          frame "氨氮" {
            w195 = u16 3 items=["总磷"=1, "总氮"=2, "氨氮"=3, "CODMn"=21, "CODcr"=22] ("站号")
            n94 = call-poly "获取测试数据.vi"("站号"=w195) -> ("测量数据区"=w196:T16)  [unwired: 10 in]
            n95 = Unbundle By Name(w196) -> ("水样数据时间"=w197:timestamp, "水样实测值"=w198:sgl)
          }
          frame "总磷" {
            w199 = u16 1 items=["总磷"=1, "总氮"=2, "氨氮"=3, "CODMn"=21, "CODcr"=22] ("站号")
            n96 = call-poly "获取测试数据.vi"("站号"=w199) -> ("测量数据区"=w200:T16)  [unwired: 10 in]
            n97 = Unbundle By Name(w200) -> ("水样数据时间"=w201:timestamp, "水样实测值"=w202:sgl)
          }
          frame "总氮" {
            w203 = u16 2 items=["总磷"=1, "总氮"=2, "氨氮"=3, "CODMn"=21, "CODcr"=22] ("站号")
            n98 = call-poly "获取测试数据.vi"("站号"=w203) -> ("测量数据区"=w204:T16)  [unwired: 10 in]
            n99 = Unbundle By Name(w204) -> ("水样数据时间"=w205:timestamp, "水样实测值"=w206:sgl)
          }
          frame "CODMn" {
            w207 = u16 21 items=["总磷"=1, "总氮"=2, "氨氮"=3, "CODMn"=21, "CODcr"=22] ("站号")
            n100 = call-poly "获取测试数据.vi"("站号"=w207) -> ("测量数据区"=w208:T16)  [unwired: 10 in]
            n101 = Unbundle By Name(w208) -> ("水样数据时间"=w209:timestamp, "水样实测值"=w210:sgl)
          }
          frame "CODCr" {
            w211 = u16 22 items=["总磷"=1, "总氮"=2, "氨氮"=3, "CODMn"=21, "CODcr"=22] ("站号")
            n102 = call-poly "获取测试数据.vi"("站号"=w211) -> ("测量数据区"=w212:T16)  [unwired: 10 in]
            n103 = Unbundle By Name(w212) -> ("水样数据时间"=w213:timestamp, "水样实测值"=w214:sgl)
          }
        }
        n104 = property class="Clust (严格)"(reference=w157) -> (reference out=w158:refnum<vi>, "Value"=w159:T2)  [unwired: 1 in, 1 out]
        n105 = property class="Clust (严格)"(reference=w188) -> (reference out=w187:refnum<vi>, "Value"=w186:T5)  [unwired: 1 in, 1 out]
        n106 = Index Array(array=w174, index=9 ("索引")) -> (element=w175:refnum<vi>)
        n107 = property class="DigNum (严格)"(reference=w175) -> (reference out=w173:refnum<vi>, "Value"=w172:u16)  [unwired: 1 in, 1 out]
        n108 = Increment(x=w172) -> (x+1=w171:u16)
        n109 = property class="DigNum (严格)"(reference=w173, "Value"=w171) -> ()  [unwired: 1 in, 2 out]
        n110 = Less Or Equal?(x=w171, y=u16 5) -> (x <= y?=w169:bool)
        n111 = Select(t=w168, s=w169, f="exit") -> (s? t:f=w166:string)
        n112 = local write "水样测试时间"(w156) -> ()
        n113 = local read "水样测试启动时间"() -> (w184:timestamp)
        n114 = Subtract(x=w156, y=w184) -> (x-y=w183:dbl)
        n115 = Bundle By Name(cluster=w162, "时间"=w156, "第一次水样浓度值"=w155) -> (w161:T15)
        n116 = Bundle By Name(cluster=w159, "时间"=w156, "集成干预测试浓度值"=w155) -> (w160:T2)
        n117 = Bundle By Name(cluster=w186, "加标前水样浓度"=w155) -> (w185:T5)
        n118 = Absolute Value(x=w183) -> (abs(x)=w182:dbl)
        n119 = property class="Clust (严格)"(reference=w164, "Value"=w161) -> ()  [unwired: 1 in, 2 out]
        n120 = property class="Clust (严格)"(reference=w158, "Value"=w160) -> ()  [unwired: 1 in, 2 out]
        n121 = property class="Clust (严格)"(reference=w187, "Value"=w185) -> ()  [unwired: 1 in, 2 out]
        n122 = Less?(x=w182, y=300.0) -> (x < y?=w178:bool)
        n123 = case shown="假" w178 {
          tunnel: w177 -> [w192 _]
          frame False {
            w191 = "获取水样数据异常" ("日志信息")
            n124 = call "启动日志.vi"("日志信息"=w191, "Slave ID"=w192) -> ()  [unwired: 9 in, 1 out]
            n125 = call "报警信息记录.vi"("报警信息"=w191, "Slave ID"=w192) -> ()  [unwired: 9 in, 1 out]
          }
          frame True {
          }
        }
        n126 = Select(t="", s=w178, f=w166) -> (s? t:f=w179:string)
        n127 = call "Add State to Queue.vi"("State(s) In Front (\"\")"=w179, "State(s) In (\"\")"=w190) -> ("States Out"=w189:string)  [unwired: 13 in]
      }
      frame "获取集成干预前测试数据" {
        n128 = call "启动日志.vi"("日志信息"=w225, "Slave ID"=w219) -> ()  [unwired: 9 in, 1 out]
        n129 = property class="Clust (严格)"(reference=w220) -> (reference out=w221:refnum<vi>, "Value"=w222:T2)  [unwired: 1 in, 1 out]
        n130 = case shown="\"CODMn\"" w219 {
          tunnel: ["" "氨氮" "总磷" "总氮" "CODMn" "CODCr"] -> w218
          frame "null", Default {
          }
          frame "氨氮" {
          }
          frame "总磷" {
          }
          frame "总氮" {
          }
          frame "CODMn" {
          }
          frame "CODCr" {
          }
        }
        n131 = call "Add State to Queue.vi"("State(s) In (\"\")"=w227) -> ("States Out"=w226:string)  [unwired: 14 in]
        n132 = call "获取最新一笔数据.vi"("table"=w218) -> ("检测值"=w217:cluster{"时间":timestamp, "检测值":dbl})  [unwired: 8 in, 2 out]
        n133 = Unbundle By Name(w217) -> ("时间"=w216:timestamp, "检测值"=w215:dbl)
        n134 = Bundle By Name(cluster=w222, "集成干预前测试时间"=w216, "集成干预前测试浓度值"=w215) -> (w223:T2)
        n135 = property class="Clust (严格)"(reference=w221, "Value"=w223) -> ()  [unwired: 1 in, 2 out]
      }
      frame "获取加标回收测试数据" {
        n136 = call "启动日志.vi"("日志信息"=w235, "Slave ID"=w246) -> ()  [unwired: 9 in, 1 out]
        n137 = case shown="\"CODCr\"" w246 {
          tunnel: [sgl 0.0 ("水样实测值") w269 w273 w277 w281 w285] -> w255
          tunnel: [timestamp(0 s since 1904-01-01) ("加标回收数据时间") w268 w272 w276 w280 w284] -> w252
          frame "null", Default {
          }
          frame "氨氮" {
            w266 = u16 3 items=["总磷"=1, "总氮"=2, "氨氮"=3, "CODMn"=21, "CODcr"=22] ("站号")
            n138 = call-poly "获取测试数据.vi"("站号"=w266) -> ("测量数据区"=w267:T17)  [unwired: 10 in]
            n139 = Unbundle By Name(w267) -> ("加标回收数据时间"=w268:timestamp, "加标回收实测值"=w269:sgl)
          }
          frame "总磷" {
            w270 = u16 1 items=["总磷"=1, "总氮"=2, "氨氮"=3, "CODMn"=21, "CODcr"=22] ("站号")
            n140 = call-poly "获取测试数据.vi"("站号"=w270) -> ("测量数据区"=w271:T17)  [unwired: 10 in]
            n141 = Unbundle By Name(w271) -> ("加标回收数据时间"=w272:timestamp, "加标回收实测值"=w273:sgl)
          }
          frame "总氮" {
            w274 = u16 2 items=["总磷"=1, "总氮"=2, "氨氮"=3, "CODMn"=21, "CODcr"=22] ("站号")
            n142 = call-poly "获取测试数据.vi"("站号"=w274) -> ("测量数据区"=w275:T17)  [unwired: 10 in]
            n143 = Unbundle By Name(w275) -> ("加标回收数据时间"=w276:timestamp, "加标回收实测值"=w277:sgl)
          }
          frame "CODMn" {
            w278 = u16 21 items=["总磷"=1, "总氮"=2, "氨氮"=3, "CODMn"=21, "CODcr"=22] ("站号")
            n144 = call-poly "获取测试数据.vi"("站号"=w278) -> ("测量数据区"=w279:T17)  [unwired: 10 in]
            n145 = Unbundle By Name(w279) -> ("加标回收数据时间"=w280:timestamp, "加标回收实测值"=w281:sgl)
          }
          frame "CODCr" {
            w282 = u16 22 items=["总磷"=1, "总氮"=2, "氨氮"=3, "CODMn"=21, "CODcr"=22] ("站号")
            n146 = call-poly "获取测试数据.vi"("站号"=w282) -> ("测量数据区"=w283:T17)  [unwired: 10 in]
            n147 = Unbundle By Name(w283) -> ("加标回收数据时间"=w284:timestamp, "加标回收实测值"=w285:sgl)
          }
        }
        n148 = property class="Clust (严格)"(reference=w259) -> (reference out=w258:refnum<vi>, "Value"=w257:T5)  [unwired: 1 in, 1 out]
        n149 = Index Array(array=w237, index=10 ("索引")) -> (element=w245:refnum<vi>)
        n150 = property class="DigNum (严格)"(reference=w245) -> (reference out=w243:refnum<vi>, "Value"=w242:u16)  [unwired: 1 in, 1 out]
        n151 = Increment(x=w242) -> (x+1=w241:u16)
        n152 = property class="DigNum (严格)"(reference=w243, "Value"=w241) -> ()  [unwired: 1 in, 2 out]
        n153 = Less Or Equal?(x=w241, y=u16 5) -> (x <= y?=w239:bool)
        n154 = Select(t=w235, s=w239, f="exit") -> (s? t:f=w236:string)
        n155 = local write "加标回收测试时间"(w252) -> ()
        n156 = local read "加标回收启动时间"() -> (w253:timestamp)
        n157 = Subtract(x=w252, y=w253) -> (x-y=w251:dbl)
        n158 = Bundle By Name(cluster=w257, "加标后水样浓度"=w255) -> (w256:T5)
        n159 = Absolute Value(x=w251) -> (abs(x)=w248:dbl)
        n160 = property class="Clust (严格)"(reference=w258, "Value"=w256) -> ()  [unwired: 1 in, 2 out]
        n161 = Less?(x=w248, y=300.0) -> (x < y?=w247:bool)
        n162 = case shown="假" w247 {
          tunnel: w246 -> [w263 _]
          frame False {
            w262 = "获取加标数据异常" ("日志信息")
            n163 = call "启动日志.vi"("日志信息"=w262, "Slave ID"=w263) -> ()  [unwired: 9 in, 1 out]
            n164 = call "报警信息记录.vi"("报警信息"=w262, "Slave ID"=w263) -> ()  [unwired: 9 in, 1 out]
          }
          frame True {
          }
        }
        n165 = Select(t="", s=w247, f=w236) -> (s? t:f=w249:string)
        n166 = call "Add State to Queue.vi"("State(s) In Front (\"\")"=w249, "State(s) In (\"\")"=w261) -> ("States Out"=w260:string)  [unwired: 13 in]
      }
      frame "获取平行样测试数据" {
        n167 = call "启动日志.vi"("日志信息"=w289, "Slave ID"=w300) -> ()  [unwired: 9 in, 1 out]
        n168 = property class="Clust (严格)"(reference=w287) -> (reference out=w311:refnum<vi>, "Value"=w310:T15)  [unwired: 1 in, 1 out]
        n169 = case shown="\"CODCr\"" w300 {
          tunnel: [sgl 0.0 ("水样实测值") w321 w325 w329 w333 w337] -> w308
          tunnel: [timestamp(0 s since 1904-01-01) ("加标回收数据时间") w320 w324 w328 w332 w336] -> w286
          frame "null", Default {
          }
          frame "氨氮" {
            w318 = u16 3 items=["总磷"=1, "总氮"=2, "氨氮"=3, "CODMn"=21, "CODcr"=22] ("站号")
            n170 = call-poly "获取测试数据.vi"("站号"=w318) -> ("测量数据区"=w319:T16)  [unwired: 10 in]
            n171 = Unbundle By Name(w319) -> ("水样数据时间"=w320:timestamp, "水样实测值"=w321:sgl)
          }
          frame "总磷" {
            w322 = u16 1 items=["总磷"=1, "总氮"=2, "氨氮"=3, "CODMn"=21, "CODcr"=22] ("站号")
            n172 = call-poly "获取测试数据.vi"("站号"=w322) -> ("测量数据区"=w323:T16)  [unwired: 10 in]
            n173 = Unbundle By Name(w323) -> ("水样数据时间"=w324:timestamp, "水样实测值"=w325:sgl)
          }
          frame "总氮" {
            w326 = u16 2 items=["总磷"=1, "总氮"=2, "氨氮"=3, "CODMn"=21, "CODcr"=22] ("站号")
            n174 = call-poly "获取测试数据.vi"("站号"=w326) -> ("测量数据区"=w327:T16)  [unwired: 10 in]
            n175 = Unbundle By Name(w327) -> ("水样数据时间"=w328:timestamp, "水样实测值"=w329:sgl)
          }
          frame "CODMn" {
            w330 = u16 21 items=["总磷"=1, "总氮"=2, "氨氮"=3, "CODMn"=21, "CODcr"=22] ("站号")
            n176 = call-poly "获取测试数据.vi"("站号"=w330) -> ("测量数据区"=w331:T16)  [unwired: 10 in]
            n177 = Unbundle By Name(w331) -> ("水样数据时间"=w332:timestamp, "水样实测值"=w333:sgl)
          }
          frame "CODCr" {
            w334 = u16 22 items=["总磷"=1, "总氮"=2, "氨氮"=3, "CODMn"=21, "CODcr"=22] ("站号")
            n178 = call-poly "获取测试数据.vi"("站号"=w334) -> ("测量数据区"=w335:T16)  [unwired: 10 in]
            n179 = Unbundle By Name(w335) -> ("水样数据时间"=w336:timestamp, "水样实测值"=w337:sgl)
          }
        }
        n180 = Index Array(array=w291, index=10 ("索引")) -> (element=w299:refnum<vi>)
        n181 = property class="DigNum (严格)"(reference=w299) -> (reference out=w297:refnum<vi>, "Value"=w296:u16)  [unwired: 1 in, 1 out]
        n182 = Increment(x=w296) -> (x+1=w295:u16)
        n183 = property class="DigNum (严格)"(reference=w297, "Value"=w295) -> ()  [unwired: 1 in, 2 out]
        n184 = Less Or Equal?(x=w295, y=u16 5) -> (x <= y?=w293:bool)
        n185 = Select(t=w289, s=w293, f="exit") -> (s? t:f=w290:string)
        n186 = Bundle By Name(cluster=w310, "第二次水样测试时间"=w286, "第二次水样浓度值"=w308) -> (w309:T15)
        n187 = local read "平行样启动时间"() -> (w306:timestamp)
        n188 = Subtract(x=w286, y=w306) -> (x-y=w305:dbl)
        n189 = property class="Clust (严格)"(reference=w311, "Value"=w309) -> ()  [unwired: 1 in, 2 out]
        n190 = Absolute Value(x=w305) -> (abs(x)=w302:dbl)
        n191 = Less?(x=w302, y=300.0) -> (x < y?=w301:bool)
        n192 = case shown="假" w301 {
          tunnel: w300 -> [w315 _]
          frame False {
            w314 = "获取平行样数据异常" ("日志信息")
            n193 = call "启动日志.vi"("日志信息"=w314, "Slave ID"=w315) -> ()  [unwired: 9 in, 1 out]
            n194 = call "报警信息记录.vi"("报警信息"=w314, "Slave ID"=w315) -> ()  [unwired: 9 in, 1 out]
          }
          frame True {
          }
        }
        n195 = Select(t="", s=w301, f=w290) -> (s? t:f=w303:string)
        n196 = call "Add State to Queue.vi"("State(s) In Front (\"\")"=w303, "State(s) In (\"\")"=w313) -> ("States Out"=w312:string)  [unwired: 13 in]
      }
      frame "计算加标体积" {
        n197 = call "启动日志.vi"("日志信息"=w340, "Slave ID"=w339) -> ()  [unwired: 9 in, 1 out]
        n198 = property class="Clust (严格)"(reference=w346) -> (reference out=w345:refnum<vi>, "Value"=w344:T5)  [unwired: 1 in, 1 out]
        n199 = call "加标回收率计算.vi"("参数"=w344) -> ("参数 out"=w343:T5)  [unwired: 9 in, 1 out]
        n200 = Bundle By Name(cluster=w343, "加标回收率"=0.0) -> (w342:T5)
        n201 = property class="Clust (严格)"(reference=w345, "Value"=w342) -> ()  [unwired: 1 in, 2 out]
        n202 = call "Add State to Queue.vi"("State(s) In (\"\")"=w348) -> ("States Out"=w347:string)  [unwired: 14 in]
      }
      frame "计算加标回收率" {
        n203 = call "启动日志.vi"("日志信息"=w350, "Slave ID"=w351) -> ()  [unwired: 9 in, 1 out]
        n204 = property class="Clust (严格)"(reference=w355) -> (reference out=w354:refnum<vi>, "Value"=w353:T5)  [unwired: 1 in, 1 out]
        n205 = call "加标回收率计算.vi"("参数"=w353) -> ("参数 out"=w352:T5)  [unwired: 9 in, 1 out]
        n206 = property class="Clust (严格)"(reference=w354, "Value"=w352) -> ()  [unwired: 1 in, 2 out]
        n207 = call "Add State to Queue.vi"("State(s) In (\"\")"=w357) -> ("States Out"=w356:string)  [unwired: 14 in]
      }
      frame "存储加标回收测试数据" {
        n208 = call "启动日志.vi"("日志信息"=w361, "Slave ID"=w362) -> ()  [unwired: 9 in, 1 out]
        n209 = case shown="\"总氮\"" w362 {
          tunnel: ["" "氨氮加标回收率" "总磷加标回收率" "总氮加标回收率" "CODMn加标回收率" "CODCr加标回收率"] -> w363
          frame "null", Default {
          }
          frame "氨氮" {
          }
          frame "总磷" {
          }
          frame "总氮" {
          }
          frame "CODMn" {
          }
          frame "CODCr" {
          }
        }
        n210 = property class="Clust (严格)"(reference=w373) -> ("Value"=w370:T5)  [unwired: 1 in, 2 out]
        n211 = Unbundle By Name(w370) -> ("加标前水样浓度"=w369:dbl, "加标后水样浓度"=w368:dbl, "加标母液浓度"=w367:dbl, "加标体积"=w366:dbl, "加标水杯定容体积"=w365:dbl, "加标回收率"=w364:dbl)
        n212 = call "Add State to Queue.vi"("State(s) In (\"\")"=w375) -> ("States Out"=w374:string)  [unwired: 14 in]
        n213 = Bundle By Name(cluster=T8 {"时间"=timestamp(0 s since 1904-01-01), "参数"="", "数据类型"="N", "加标回收率"=0.0, "加标前水样测试时间"=timestamp(0 s since 1904-01-01), "加标前水样浓度值"=0.0, "加标后水样浓度值"=0.0, "加标母液浓度值"=0.0, "加标体积"=0.0, "加标水杯定容体积"=0.0} ("data in"), "时间"="加标回收测试时间", "参数"=w363, "加标前水样测试时间"="水样测试时间", "加标前水样浓度值"=w369, "加标后水样浓度值"=w368, "加标母液浓度值"=w367, "加标体积"=w366, "加标水杯定容体积"=w365, "加标回收率"=w364) -> (w359:T8)
        n214 = call "加标回收数据插入.vi"("data in"=w359) -> ()  [unwired: 10 in, 1 out]
      }
      frame "存储平行样测试数据" {
        n215 = call "启动日志.vi"("日志信息"=w388, "Slave ID"=w389) -> ()  [unwired: 9 in, 1 out]
        n216 = property class="Clust (严格)"(reference=w386) -> (reference out=w384:refnum<vi>, "Value"=w385:T15)  [unwired: 1 in, 1 out]
        n217 = case shown="\"CODMn\"" w389 {
          tunnel: ["" "氨氮" "总磷" "总氮" "CODMn" "CODCr"] -> w382
          frame "null", Default {
          }
          frame "氨氮" {
          }
          frame "总磷" {
          }
          frame "总氮" {
          }
          frame "CODMn" {
          }
          frame "CODCr" {
          }
        }
        n218 = call "Add State to Queue.vi"("State(s) In (\"\")"=w391) -> ("States Out"=w390:string)  [unwired: 14 in]
        n219 = Bundle By Name(cluster=w385, "参数"=w382) -> (w383:T15)
        n220 = property class="Clust (严格)"(reference=w384, "Value"=w383) -> ()  [unwired: 1 in, 2 out]
        n221 = call "平行样数据插入.vi"("平行样测试数据"=w383) -> ()  [unwired: 10 in, 1 out]
      }
      frame "存储集成干预测试数据" {
        n222 = call "启动日志.vi"("日志信息"=w405, "Slave ID"=w400) -> ()  [unwired: 9 in, 1 out]
        n223 = property class="Clust (严格)"(reference=w403) -> (reference out=w401:refnum<vi>, "Value"=w402:T2)  [unwired: 1 in, 1 out]
        n224 = case shown="\"CODMn\"" w400 {
          tunnel: ["" "氨氮" "总磷" "总氮" "CODMn" "CODCr"] -> w399
          frame "null", Default {
          }
          frame "氨氮" {
          }
          frame "总磷" {
          }
          frame "总氮" {
          }
          frame "CODMn" {
          }
          frame "CODCr" {
          }
        }
        n225 = call "Add State to Queue.vi"("State(s) In (\"\")"=w407) -> ("States Out"=w406:string)  [unwired: 14 in]
        n226 = Bundle By Name(cluster=w402, "参数"=w399) -> (w398:T2)
        n227 = property class="Clust (严格)"(reference=w401, "Value"=w398) -> ()  [unwired: 1 in, 2 out]
        n228 = call "集成干预数据插入.vi"("集成干预测试数据"=w398) -> ()  [unwired: 10 in, 1 out]
      }
      frame "流程结束" {
        n229 = global read "ZK非断电保存全局变量.vi" "流程运行状态标记位"() -> (w420:T7)
        n230 = case shown="\"CODCr\"" w418 {
          tunnel: "空闲" -> [_ w424 w425 w426 w427 w428]
          frame "null", Default {
          }
          frame "氨氮" {
            n231 = global write "ZK非断电保存全局变量.vi" "氨氮加标模块运行状态"(w424) -> ()
          }
          frame "总磷" {
            n232 = global write "ZK非断电保存全局变量.vi" "总磷加标模块运行状态"(w425) -> ()
          }
          frame "总氮" {
            n233 = global write "ZK非断电保存全局变量.vi" "总氮加标模块运行状态"(w426) -> ()
          }
          frame "CODMn" {
            n234 = global write "ZK非断电保存全局变量.vi" "CODMn加标模块运行状态"(w427) -> ()
          }
          frame "CODCr" {
            n235 = global write "ZK非断电保存全局变量.vi" "CODcr加标模块运行状态"(w428) -> ()
          }
        }
        n236 = Concatenate Strings("----->>" ("字符串"), w417) -> (w416:string)
        n237 = case shown="\"总磷\"" w418 {
          tunnel: w420 -> [_ w431 w432 w435 w438 w441]
          frame "null", Default {
          }
          frame "氨氮" {
            n238 = Bundle By Name(cluster=w431, "氨氮"=FALSE) -> (w430:T7)
            n239 = global write "ZK非断电保存全局变量.vi" "流程运行状态标记位"(w430) -> ()
          }
          frame "总磷" {
            n240 = Bundle By Name(cluster=w432, "总磷"=FALSE ("氨氮")) -> (w434:T7)
            n241 = global write "ZK非断电保存全局变量.vi" "流程运行状态标记位"(w434) -> ()
          }
          frame "总氮" {
            n242 = Bundle By Name(cluster=w435, "总氮"=FALSE ("氨氮")) -> (w437:T7)
            n243 = global write "ZK非断电保存全局变量.vi" "流程运行状态标记位"(w437) -> ()
          }
          frame "CODMn" {
            n244 = Bundle By Name(cluster=w438, "CODMn"=FALSE ("氨氮")) -> (w440:T7)
            n245 = global write "ZK非断电保存全局变量.vi" "流程运行状态标记位"(w440) -> ()
          }
          frame "CODCr" {
            n246 = Bundle By Name(cluster=w441, "CODCr"=FALSE ("氨氮")) -> (w443:T7)
            n247 = global write "ZK非断电保存全局变量.vi" "流程运行状态标记位"(w443) -> ()
          }
        }
        n248 = call "启动日志.vi"("日志信息"=w416, "Slave ID"=w418) -> ()  [unwired: 9 in, 1 out]
        n249 = call "Add State to Queue.vi"("State(s) In (\"\")"=w423) -> ("States Out"=w422:string)  [unwired: 14 in]
      }
      frame "流程退出" {
        n250 = Concatenate Strings("----->>" ("字符串"), w447) -> (w446:string)
        n251 = call "启动日志.vi"("日志信息"=w446, "Slave ID"=w448) -> ()  [unwired: 9 in, 1 out]
        n252 = call "Add State to Queue.vi"("State(s) In (\"\")"=w451) -> ("States Out"=w450:string)  [unwired: 14 in]
      }
      frame "-------------------# 采配水流程 #-------------------" {
        n253 = call "Add State to Queue.vi"("State(s) In (\"\")"=w454) -> ("States Out"=w453:string)  [unwired: 14 in]
      }
      frame "采水单元启动水样测试流程" {
        n254 = call "启动日志.vi"("日志信息"=w457, "Slave ID"=w458) -> ()  [unwired: 9 in, 1 out]
        n255 = call "采配水启动器.vi"("启动/停止命令"=T9."水样测试（全流程）") -> ()  [unwired: 10 in, 1 out]
        n256 = Index Array(array=w463) -> (element=w462:refnum<vi>)  [unwired: 1 in]
        n257 = property class="DigNum (严格)"(reference=w462) -> (reference out=w461:refnum<vi>, "Value"=w460:u16)  [unwired: 1 in, 1 out]
        n258 = Increment(x=w460) -> (x+1=w459:u16)
        n259 = property class="DigNum (严格)"(reference=w461, "Value"=w459) -> ()  [unwired: 1 in, 2 out]
        n260 = call "Add State to Queue.vi"("State(s) In (\"\")"=w465) -> ("States Out"=w464:string)  [unwired: 14 in]
      }
      frame "采水单元启动加标回收流程" {
        n261 = call "启动日志.vi"("日志信息"=w468, "Slave ID"=w469) -> ()  [unwired: 9 in, 1 out]
        n262 = call "采配水启动器.vi"("启动/停止命令"=T9."加标回收") -> ()  [unwired: 10 in, 1 out]
        n263 = Index Array(array=w474) -> (element=w473:refnum<vi>)  [unwired: 1 in]
        n264 = property class="DigNum (严格)"(reference=w473) -> (reference out=w472:refnum<vi>, "Value"=w471:u16)  [unwired: 1 in, 1 out]
        n265 = Increment(x=w471) -> (x+1=w470:u16)
        n266 = property class="DigNum (严格)"(reference=w472, "Value"=w470) -> ()  [unwired: 1 in, 2 out]
        n267 = call "Add State to Queue.vi"("State(s) In (\"\")"=w476) -> ("States Out"=w475:string)  [unwired: 14 in]
      }
      frame "判断采水单元水样测试流程是否启动" {
        n268 = call "启动日志.vi"("日志信息"=w480, "Slave ID"=w479) -> ()  [unwired: 9 in, 1 out]
        n269 = call "获取采配水运行状态.vi"() -> ("运行流程"=w493:T11)  [unwired: 10 in, 1 out]
        n270 = Equal?(x=T10."待机" ("运行流程"), y=w493) -> (x = y?=w492:bool)
        n271 = Index Array(array=w484, index=0 ("索引")) -> (element=w483:refnum<vi>)
        n272 = property class="DigNum (严格)"(reference=w483) -> ("Value"=w482:u16)  [unwired: 1 in, 2 out]
        n273 = Greater Or Equal?(x=w482, y=u16 5) -> (x >= y?=w478:bool)
        n274 = Select(t="采水单元启动水样测试流程\n判断采水单元水样测试流程是否启动" ("State(s) In (\"\")"), s=w492, f="") -> (s? t:f=w487:string)
        n275 = case shown="真" w478 {
          tunnel: w479 -> [_ w497]
          frame False {
          }
          frame True {
            w496 = "采水单元启动失败" ("日志信息")
            n276 = call "启动日志.vi"("日志信息"=w496, "Slave ID"=w497) -> ()  [unwired: 9 in, 1 out]
            n277 = call "报警信息记录.vi"("报警信息"=w496, "Slave ID"=w497) -> ()  [unwired: 9 in, 1 out]
          }
        }
        n278 = Select(t="流程结束" ("State(s) In (\"\")"), s=w478, f=w487) -> (s? t:f=w486:string)
        n279 = call "Add State to Queue.vi"("State(s) In Front (\"\")"=w486, "State(s) In (\"\")"=w495) -> ("States Out"=w494:string)  [unwired: 13 in]
      }
      frame "判断采水单元加标回收流程是否启动" {
        n280 = call "启动日志.vi"("日志信息"=w501, "Slave ID"=w500) -> ()  [unwired: 9 in, 1 out]
        n281 = call "获取采配水运行状态.vi"() -> ("运行流程"=w515:T11)  [unwired: 10 in, 1 out]
        n282 = Equal?(x=T10."待机" ("运行流程"), y=w515) -> (x = y?=w514:bool)
        n283 = Index Array(array=w506, index=0 ("索引")) -> (element=w505:refnum<vi>)
        n284 = property class="DigNum (严格)"(reference=w505) -> ("Value"=w504:u16)  [unwired: 1 in, 2 out]
        n285 = Greater Or Equal?(x=w504, y=u16 5) -> (x >= y?=w499:bool)
        n286 = Select(t="采水单元启动加标回收流程\n判断采水单元加标回收流程是否启动" ("State(s) In (\"\")"), s=w514, f="") -> (s? t:f=w509:string)
        n287 = case shown="真" w499 {
          tunnel: w500 -> [_ w518]
          frame False {
          }
          frame True {
            w517 = "采水单元启动失败" ("日志信息")
            n288 = call "启动日志.vi"("日志信息"=w517, "Slave ID"=w518) -> ()  [unwired: 9 in, 1 out]
            n289 = call "报警信息记录.vi"("报警信息"=w517, "Slave ID"=w518) -> ()  [unwired: 9 in, 1 out]
          }
        }
        n290 = Select(t="流程结束" ("State(s) In (\"\")"), s=w499, f=w509) -> (s? t:f=w508:string)
        n291 = call "Add State to Queue.vi"("State(s) In Front (\"\")"=w508, "State(s) In (\"\")"=w502) -> ("States Out"=w516:string)  [unwired: 13 in]
      }
      frame "采水单元润洗" {
        n292 = call "获取采配水运行状态.vi"() -> ("运行流程"=w529:T11)  [unwired: 10 in, 1 out]
        n293 = Equal To 0?(x=w529) -> (x = 0?=w521:bool)
        n294 = Less?(x=w529, y=T10."采样" ("运行流程")) -> (x < y?=w532:bool)
        n295 = Greater?(x=w529, y=T10."待机" ("运行流程")) -> (0:w533:bool)
        n296 = case shown="真" w519 {
          tunnel: w522 -> [_ w539]
          tunnel: w523 -> [_ w538]
          frame False {
          }
          frame True {
            n297 = call "启动日志.vi"("日志信息"=w538, "Slave ID"=w539) -> ()  [unwired: 9 in, 1 out]
          }
        }
        n298 = And(x=w532, y=w533) -> (x .and. y?=w531:bool)
        n299 = case shown="真" w521 {
          tunnel: w522 -> [_ w537]
          frame False {
          }
          frame True {
            w536 = "采水单元流程中断" ("日志信息")
            n300 = call "启动日志.vi"("日志信息"=w536, "Slave ID"=w537) -> ()  [unwired: 9 in, 1 out]
            n301 = call "报警信息记录.vi"("报警信息"=w536, "Slave ID"=w537) -> ()  [unwired: 9 in, 1 out]
          }
        }
        n302 = Select(t=w523, s=w531, f="") -> (s? t:f=w527:string)
        n303 = Select(t="流程结束" ("State(s) In (\"\")"), s=w521, f=w527) -> (s? t:f=w526:string)
        n304 = call "Add State to Queue.vi"("State(s) In Front (\"\")"=w526, "State(s) In (\"\")"=w535) -> ("States Out"=w534:string)  [unwired: 13 in]
      }
      frame "采水单元采样" {
        n305 = call "获取采配水运行状态.vi"() -> ("运行流程"=w546:T11)  [unwired: 10 in, 1 out]
        n306 = Equal To 0?(x=w546) -> (x = 0?=w543:bool)
        n307 = Equal?(x=T10."采样" ("运行流程"), y=w546) -> (x = y?=w545:bool)
        n308 = case shown="真" w540 {
          tunnel: w542 -> [_ w557]
          tunnel: w544 -> [_ w556]
          frame False {
          }
          frame True {
            n309 = call "启动日志.vi"("日志信息"=w556, "Slave ID"=w557) -> ()  [unwired: 9 in, 1 out]
          }
        }
        n310 = case shown="真" w543 {
          tunnel: w542 -> [_ w555]
          frame False {
          }
          frame True {
            w554 = "采水单元流程中断" ("日志信息")
            n311 = call "启动日志.vi"("日志信息"=w554, "Slave ID"=w555) -> ()  [unwired: 9 in, 1 out]
            n312 = call "报警信息记录.vi"("报警信息"=w554, "Slave ID"=w555) -> ()  [unwired: 9 in, 1 out]
          }
        }
        n313 = Select(t=w544, s=w545, f="") -> (s? t:f=w549:string)
        n314 = Select(t="流程结束" ("State(s) In (\"\")"), s=w543, f=w549) -> (s? t:f=w548:string)
        n315 = call "Add State to Queue.vi"("State(s) In Front (\"\")"=w548, "State(s) In (\"\")"=w553) -> ("States Out"=w552:string)  [unwired: 13 in]
      }
      frame "水样沉淀" {
        n316 = global read "系统交互.vi" "站点类型"() -> (w563:enum16{"一体站", "固定站", "浮船", "一体站V1-V3"})
        n317 = case shown="真" w559 {
          tunnel: w562 -> [_ w581]
          tunnel: w565 -> [_ w580]
          frame False {
          }
          frame True {
            n318 = call "启动日志.vi"("日志信息"=w580, "Slave ID"=w581) -> ()  [unwired: 9 in, 1 out]
          }
        }
        n319 = case shown="\"浮船\"" w563 {
          tunnel: [w577 _ _] -> w564
          tunnel: w559 -> [w576 _ _]
          frame "一体站", Default {
            n320 = case shown="真" w576 {
              tunnel: [_ w578] -> w577
              frame False {
              }
              frame True {
                n321 = call "质控模块润洗OK命令.vi"("质控润洗OK"=TRUE) -> ("error out"=w578:errorcluster)  [unwired: 10 in]
              }
            }
          }
          frame "固定站" {
          }
          frame "浮船" {
          }
        }
        n322 = call "获取采配水运行状态.vi"("error in (no error)"=w564) -> ("运行流程"=w569:T11)  [unwired: 9 in, 1 out]
        n323 = Equal To 0?(x=w569) -> (x = 0?=w561:bool)
        n324 = Equal?(x=采配水通用流程."沉淀" ("运行流程"), y=w569) -> (x = y?=w571:bool)
        n325 = case shown="真" w561 {
          tunnel: w562 -> [_ w575]
          frame False {
          }
          frame True {
            w574 = "采水单元流程中断" ("日志信息")
            n326 = call "启动日志.vi"("日志信息"=w574, "Slave ID"=w575) -> ()  [unwired: 9 in, 1 out]
            n327 = call "报警信息记录.vi"("报警信息"=w574, "Slave ID"=w575) -> ()  [unwired: 9 in, 1 out]
          }
        }
        n328 = Select(t=w565, s=w571, f="") -> (s? t:f=w567:string)
        n329 = Select(t="流程结束" ("State(s) In (\"\")"), s=w561, f=w567) -> (s? t:f=w566:string)
        n330 = call "Add State to Queue.vi"("State(s) In Front (\"\")"=w566, "State(s) In (\"\")"=w573) -> ("States Out"=w572:string)  [unwired: 13 in]
      }
      frame "水样配水" {
        n331 = call "获取采配水运行状态.vi"() -> ("运行流程"=w592:T11)  [unwired: 10 in, 1 out]
        n332 = Equal To 0?(x=w592) -> (x = 0?=w586:bool)
        n333 = Equal?(x=采配水通用流程."配水" ("运行流程"), y=w592) -> (x = y?=w593:bool)
        n334 = case shown="真" w583 {
          tunnel: w585 -> [_ w599]
          tunnel: w587 -> [_ w598]
          frame False {
          }
          frame True {
            n335 = call "启动日志.vi"("日志信息"=w598, "Slave ID"=w599) -> ()  [unwired: 9 in, 1 out]
          }
        }
        n336 = case shown="真" w586 {
          tunnel: w585 -> [_ w597]
          frame False {
          }
          frame True {
            w596 = "采水单元流程中断" ("日志信息")
            n337 = call "启动日志.vi"("日志信息"=w596, "Slave ID"=w597) -> ()  [unwired: 9 in, 1 out]
            n338 = call "报警信息记录.vi"("报警信息"=w596, "Slave ID"=w597) -> ()  [unwired: 9 in, 1 out]
          }
        }
        n339 = Select(t="", s=w593, f=w587) -> (s? t:f=w590:string)
        n340 = Select(t="流程结束" ("State(s) In (\"\")"), s=w586, f=w590) -> (s? t:f=w589:string)
        n341 = call "Add State to Queue.vi"("State(s) In Front (\"\")"=w589, "State(s) In (\"\")"=w595) -> ("States Out"=w594:string)  [unwired: 13 in]
      }
      frame "-------------------# 质控模块流程 #-------------------" {
        n342 = call "Add State to Queue.vi"("State(s) In (\"\")"=w602) -> ("States Out"=w601:string)  [unwired: 14 in]
      }
      frame "质控单元启动水样润洗" {
        w612 = 质控流程控制."启动水样润洗流程" ("流程控制")
        n343 = call "启动日志.vi"("日志信息"=w604, "Slave ID"=w605) -> ()  [unwired: 9 in, 1 out]
        n344 = call "ZK流程控制.vi"("流程控制"=w612, "Slave ID"=w605) -> ()  [unwired: 9 in, 1 out]
        n345 = Index Array(array=w607, index=1 ("索引")) -> (element=w611:refnum<vi>)
        n346 = property class="DigNum (严格)"(reference=w611) -> (reference out=w610:refnum<vi>, "Value"=w609:u16)  [unwired: 1 in, 1 out]
        n347 = Increment(x=w609) -> (x+1=w608:u16)
        n348 = property class="DigNum (严格)"(reference=w610, "Value"=w608) -> ()  [unwired: 1 in, 2 out]
        n349 = call "Add State to Queue.vi"("State(s) In (\"\")"=w614) -> ("States Out"=w613:string)  [unwired: 14 in]
        "加标模块润洗流程控制" <- w612
      }
      frame "质控单元启动加标润洗" {
        w616 = 质控流程控制."启动加标润洗流程" ("流程控制")
        n350 = call "启动日志.vi"("日志信息"=w617, "Slave ID"=w618) -> ()  [unwired: 9 in, 1 out]
        n351 = call "ZK流程控制.vi"("流程控制"=w616, "Slave ID"=w618) -> ()  [unwired: 9 in, 1 out]
        n352 = local write "加标模块润洗流程控制"(w616) -> ()
        n353 = Index Array(array=w620, index=7 ("索引")) -> (element=w624:refnum<vi>)
        n354 = property class="DigNum (严格)"(reference=w624) -> (reference out=w623:refnum<vi>, "Value"=w622:u16)  [unwired: 1 in, 1 out]
        n355 = Increment(x=w622) -> (x+1=w621:u16)
        n356 = property class="DigNum (严格)"(reference=w623, "Value"=w621) -> ()  [unwired: 1 in, 2 out]
        n357 = call "Add State to Queue.vi"("State(s) In (\"\")"=w626) -> ("States Out"=w625:string)  [unwired: 14 in]
      }
      frame "质控单元启动采样" {
        n358 = call "启动日志.vi"("日志信息"=w628, "Slave ID"=w629) -> ()  [unwired: 9 in, 1 out]
        n359 = call "ZK流程控制.vi"("流程控制"=质控流程控制."启动进样流程", "Slave ID"=w629) -> ()  [unwired: 9 in, 1 out]
        n360 = Index Array(array=w631, index=2 ("索引")) -> (element=w635:refnum<vi>)
        n361 = property class="DigNum (严格)"(reference=w635) -> (reference out=w634:refnum<vi>, "Value"=w633:u16)  [unwired: 1 in, 1 out]
        n362 = Increment(x=w633) -> (x+1=w632:u16)
        n363 = property class="DigNum (严格)"(reference=w634, "Value"=w632) -> ()  [unwired: 1 in, 2 out]
        n364 = call "Add State to Queue.vi"("State(s) In (\"\")"=w638) -> ("States Out"=w637:string)  [unwired: 14 in]
      }
      frame "质控单元写入加标体积" {
        n365 = call "启动日志.vi"("日志信息"=w646, "Slave ID"=w640) -> ()  [unwired: 9 in, 1 out]
        n366 = property class="Clust (严格)"(reference=w651) -> ("Value"=w650:T5)  [unwired: 1 in, 2 out]
        n367 = Index Array(array=w645, index=8 ("索引")) -> (element=w643:refnum<vi>)
        n368 = Unbundle By Name(w650) -> ("加标体积"=w649:dbl)
        n369 = property class="DigNum (严格)"(reference=w643) -> (reference out=w641:refnum<vi>, "Value"=w642:u16)  [unwired: 1 in, 1 out]
        n370 = call "ZK加标体积写入.vi"("加标体积"=w649, "Slave ID"=w640) -> ("error out"=w648:errorcluster)  [unwired: 9 in]
        n371 = case shown="错误" w648 {
          tunnel: [_ w656] -> w647
          tunnel: w646 -> [_ w658]
          tunnel: w642 -> [_ w660]
          tunnel: w641 -> [_ w662]
          tunnel: w640 -> [_ w654]
          frame No Error {
          }
          frame Error {
            n372 = Increment(x=w660) -> (x+1=w661:u16)
            n373 = Greater Or Equal?(x=w660, y=u16 5) -> (x >= y?=w655:bool)
            n374 = property class="DigNum (严格)"(reference=w662, "Value"=w661) -> ()  [unwired: 1 in, 2 out]
            n375 = case shown="真" w655 {
              tunnel: w654 -> [_ w664]
              frame False {
              }
              frame True {
                w663 = "加标体积写入异常" ("报警信息")
                n376 = call "启动日志.vi"("日志信息"=w663, "Slave ID"=w664) -> ()  [unwired: 9 in, 1 out]
                n377 = call "报警信息记录.vi"("报警信息"=w663, "Slave ID"=w664) -> ()  [unwired: 9 in, 1 out]
              }
            }
            n378 = Select(t="流程结束", s=w655, f=w658) -> (s? t:f=w656:string)
          }
        }
        n379 = call "Add State to Queue.vi"("State(s) In Front (\"\")"=w647, "State(s) In (\"\")"=w653) -> ("States Out"=w652:string)  [unwired: 13 in]
      }
      frame "质控单元启动加标" {
        n380 = call "启动日志.vi"("日志信息"=w666, "Slave ID"=w667) -> ()  [unwired: 9 in, 1 out]
        n381 = call "ZK流程控制.vi"("流程控制"=质控流程控制."启动加标流程", "Slave ID"=w667) -> ()  [unwired: 9 in, 1 out]
        n382 = Index Array(array=w670, index=3 ("索引")) -> (element=w669:refnum<vi>)
        n383 = property class="DigNum (严格)"(reference=w669) -> (reference out=w673:refnum<vi>, "Value"=w672:u16)  [unwired: 1 in, 1 out]
        n384 = Increment(x=w672) -> (x+1=w671:u16)
        n385 = property class="DigNum (严格)"(reference=w673, "Value"=w671) -> ()  [unwired: 1 in, 2 out]
        n386 = call "Add State to Queue.vi"("State(s) In (\"\")"=w676) -> ("States Out"=w675:string)  [unwired: 14 in]
      }
      frame "质控单元启动排液" {
        n387 = call "启动日志.vi"("日志信息"=w678, "Slave ID"=w679) -> ()  [unwired: 9 in, 1 out]
        n388 = call "ZK流程控制.vi"("流程控制"=质控流程控制."启动排液流程", "Slave ID"=w679) -> ()  [unwired: 9 in, 1 out]
        n389 = Index Array(array=w682, index=4 ("索引")) -> (element=w681:refnum<vi>)
        n390 = property class="DigNum (严格)"(reference=w681) -> (reference out=w685:refnum<vi>, "Value"=w684:u16)  [unwired: 1 in, 1 out]
        n391 = Increment(x=w684) -> (x+1=w683:u16)
        n392 = property class="DigNum (严格)"(reference=w685, "Value"=w683) -> ()  [unwired: 1 in, 2 out]
        n393 = call "Add State to Queue.vi"("State(s) In (\"\")"=w688) -> ("States Out"=w687:string)  [unwired: 14 in]
      }
      frame "质控单元启动搅拌" {
        n394 = call "启动日志.vi"("日志信息"=w693, "Slave ID"=w690) -> ()  [unwired: 9 in, 1 out]
        n395 = call "ZK组合命令区.vi"("是否启用通讯通知"=FALSE, "组合命令区"=质控组合命令区."进空气（搅拌）", "Slave ID"=w690) -> ()  [unwired: 8 in, 1 out]
        n396 = call "Add State to Queue.vi"("State(s) In (\"\")"=w695) -> ("States Out"=w694:string)  [unwired: 14 in]
      }
      frame "判断质控单元润洗是否启动成功" {
        n397 = local read "加标模块润洗流程控制"() -> (w704:T3)
        n398 = case shown="真" w700 {
          tunnel: w696 -> [_ w722]
          tunnel: w705 -> [_ w721]
          frame False {
          }
          frame True {
            n399 = call "启动日志.vi"("日志信息"=w722, "Slave ID"=w721) -> ()  [unwired: 9 in, 1 out]
          }
        }
        n400 = case shown="\"氨氮\"" w705 {
          tunnel: [T13."待机" ("运行状态") w728 w730 w732 w734 w736] -> w717
          frame "null", Default {
          }
          frame "氨氮" {
            n401 = global read "ZK非断电保存全局变量.vi" "氨氮质控仪器状态"() -> (w729:T18)
            n402 = Unbundle By Name(w729) -> ("运行状态"=w728:T13)
          }
          frame "总磷" {
            n403 = global read "ZK非断电保存全局变量.vi" "总磷质控仪器状态"() -> (w731:T18)
            n404 = Unbundle By Name(w731) -> ("运行状态"=w730:T13)
          }
          frame "总氮" {
            n405 = global read "ZK非断电保存全局变量.vi" "总氮质控仪器状态"() -> (w733:T18)
            n406 = Unbundle By Name(w733) -> ("运行状态"=w732:T13)
          }
          frame "CODMn" {
            n407 = global read "ZK非断电保存全局变量.vi" "CODMn质控仪器状态"() -> (w735:T18)
            n408 = Unbundle By Name(w735) -> ("运行状态"=w734:T13)
          }
          frame "CODCr" {
            n409 = global read "ZK非断电保存全局变量.vi" "CODCr质控仪器状态"() -> (w737:T18)
            n410 = Unbundle By Name(w737) -> ("运行状态"=w736:T13)
          }
        }
        n411 = case shown="\"启动水样润洗流程\", 默认" w704 {
          tunnel: ["质控单元启动水样润洗\n判断质控单元润洗是否启动成功" ("State(s) In (\"\")") "质控单元启动加标润洗\n判断质控单元润洗是否启动成功" ("State(s) In (\"\")")] -> w698
          frame "启动水样润洗流程", Default {
          }
          frame "启动加标润洗流程" {
          }
        }
        n412 = Index Array(array=w710, index=1 ("索引")) -> (element=w709:refnum<vi>)
        n413 = Greater Or Equal?(x=w703, y=10) -> (x >= y?=w699:bool)
        n414 = property class="DigNum (严格)"(reference=w709) -> ("Value"=w708:u16)  [unwired: 1 in, 2 out]
        n415 = Greater Or Equal?(x=w708, y=u16 5) -> (x >= y?=w706:bool)
        n416 = Select(t=w698, s=w699, f=w696) -> (s? t:f=w697:string)
        n417 = case shown="真" w706 {
          tunnel: w705 -> [_ w726]
          frame False {
          }
          frame True {
            w725 = "质控单元润洗启动失败" ("日志信息")
            n418 = call "启动日志.vi"("日志信息"=w725, "Slave ID"=w726) -> ()  [unwired: 9 in, 1 out]
            n419 = call "报警信息记录.vi"("报警信息"=w725, "Slave ID"=w726) -> ()  [unwired: 9 in, 1 out]
          }
        }
        n420 = Not Equal?(x=w717, y=T13."待机") -> (x != y?=w716:bool)
        n421 = And(x=w699, y=w716) -> (x .and. y?=w701:bool)
        n422 = Select(t="", s=w701, f=w697) -> (s? t:f=w714:string)
        n423 = Select(t="流程结束" ("State(s) In (\"\")"), s=w706, f=w714) -> (s? t:f=w712:string)
        n424 = call "Add State to Queue.vi"("State(s) In Front (\"\")"=w712, "State(s) In (\"\")"=w720) -> ("States Out"=w719:string)  [unwired: 13 in]
      }
      frame "判断质控单元采样是否启动成功" {
        n425 = case shown="真" w745 {
          tunnel: w739 -> [_ w763]
          tunnel: w746 -> [_ w762]
          frame False {
          }
          frame True {
            n426 = call "启动日志.vi"("日志信息"=w763, "Slave ID"=w762) -> ()  [unwired: 9 in, 1 out]
          }
        }
        n427 = case shown="\"CODCr\"" w746 {
          tunnel: [T13."待机" ("运行状态") w767 w769 w771 w773 w775] -> w758
          frame "null", Default {
          }
          frame "氨氮" {
            n428 = global read "ZK非断电保存全局变量.vi" "氨氮质控仪器状态"() -> (w768:T18)
            n429 = Unbundle By Name(w768) -> ("运行状态"=w767:T13)
          }
          frame "总磷" {
            n430 = global read "ZK非断电保存全局变量.vi" "总磷质控仪器状态"() -> (w770:T18)
            n431 = Unbundle By Name(w770) -> ("运行状态"=w769:T13)
          }
          frame "总氮" {
            n432 = global read "ZK非断电保存全局变量.vi" "总氮质控仪器状态"() -> (w772:T18)
            n433 = Unbundle By Name(w772) -> ("运行状态"=w771:T13)
          }
          frame "CODMn" {
            n434 = global read "ZK非断电保存全局变量.vi" "CODMn质控仪器状态"() -> (w774:T18)
            n435 = Unbundle By Name(w774) -> ("运行状态"=w773:T13)
          }
          frame "CODCr" {
            n436 = global read "ZK非断电保存全局变量.vi" "CODCr质控仪器状态"() -> (w776:T18)
            n437 = Unbundle By Name(w776) -> ("运行状态"=w775:T13)
          }
        }
        n438 = Index Array(array=w751, index=2 ("索引")) -> (element=w750:refnum<vi>)
        n439 = Greater Or Equal?(x=w744, y=10) -> (x >= y?=w741:bool)
        n440 = property class="DigNum (严格)"(reference=w750) -> ("Value"=w749:u16)  [unwired: 1 in, 2 out]
        n441 = Select(t="质控单元启动采样\n判断质控单元采样是否启动成功" ("State(s) In (\"\")"), s=w741, f=w739) -> (s? t:f=w738:string)
        n442 = Greater Or Equal?(x=w749, y=u16 5) -> (x >= y?=w747:bool)
        n443 = case shown="真" w747 {
          tunnel: w746 -> [_ w765]
          frame False {
          }
          frame True {
            w764 = "质控单元采样启动失败" ("日志信息")
            n444 = call "启动日志.vi"("日志信息"=w764, "Slave ID"=w765) -> ()  [unwired: 9 in, 1 out]
            n445 = call "报警信息记录.vi"("报警信息"=w764, "Slave ID"=w765) -> ()  [unwired: 9 in, 1 out]
          }
        }
        n446 = Not Equal?(x=w758, y=T13."待机") -> (x != y?=w757:bool)
        n447 = And(x=w741, y=w757) -> (x .and. y?=w742:bool)
        n448 = Select(t="", s=w742, f=w738) -> (s? t:f=w755:string)
        n449 = Select(t="流程结束" ("State(s) In (\"\")"), s=w747, f=w755) -> (s? t:f=w753:string)
        n450 = call "Add State to Queue.vi"("State(s) In Front (\"\")"=w753, "State(s) In (\"\")"=w761) -> ("States Out"=w760:string)  [unwired: 13 in]
      }
      frame "判断质控单元加标是否启动成功" {
        n451 = case shown="真" w783 {
          tunnel: w778 -> [_ w802]
          tunnel: w785 -> [_ w801]
          frame False {
          }
          frame True {
            n452 = call "启动日志.vi"("日志信息"=w802, "Slave ID"=w801) -> ()  [unwired: 9 in, 1 out]
          }
        }
        n453 = case shown="\"CODCr\"" w785 {
          tunnel: [T13."异常停机" ("运行状态") w806 w808 w810 w812 w814] -> w797
          frame "null", Default {
          }
          frame "氨氮" {
            n454 = global read "ZK非断电保存全局变量.vi" "氨氮质控仪器状态"() -> (w807:T18)
            n455 = Unbundle By Name(w807) -> ("运行状态"=w806:T13)
          }
          frame "总磷" {
            n456 = global read "ZK非断电保存全局变量.vi" "总磷质控仪器状态"() -> (w809:T18)
            n457 = Unbundle By Name(w809) -> ("运行状态"=w808:T13)
          }
          frame "总氮" {
            n458 = global read "ZK非断电保存全局变量.vi" "总氮质控仪器状态"() -> (w811:T18)
            n459 = Unbundle By Name(w811) -> ("运行状态"=w810:T13)
          }
          frame "CODMn" {
            n460 = global read "ZK非断电保存全局变量.vi" "CODMn质控仪器状态"() -> (w813:T18)
            n461 = Unbundle By Name(w813) -> ("运行状态"=w812:T13)
          }
          frame "CODCr" {
            n462 = global read "ZK非断电保存全局变量.vi" "CODCr质控仪器状态"() -> (w815:T18)
            n463 = Unbundle By Name(w815) -> ("运行状态"=w814:T13)
          }
        }
        n464 = Index Array(array=w790, index=3 ("索引")) -> (element=w789:refnum<vi>)
        n465 = Greater Or Equal?(x=w784, y=10) -> (x >= y?=w780:bool)
        n466 = property class="DigNum (严格)"(reference=w789) -> ("Value"=w788:u16)  [unwired: 1 in, 2 out]
        n467 = Select(t="质控单元启动加标\n判断质控单元加标是否启动成功" ("State(s) In (\"\")"), s=w780, f=w778) -> (s? t:f=w777:string)
        n468 = Greater Or Equal?(x=w788, y=u16 5) -> (x >= y?=w786:bool)
        n469 = case shown="真" w786 {
          tunnel: w785 -> [_ w804]
          frame False {
          }
          frame True {
            w803 = "质控单元加标启动失败" ("日志信息")
            n470 = call "启动日志.vi"("日志信息"=w803, "Slave ID"=w804) -> ()  [unwired: 9 in, 1 out]
            n471 = call "报警信息记录.vi"("报警信息"=w803, "Slave ID"=w804) -> ()  [unwired: 9 in, 1 out]
          }
        }
        n472 = Not Equal?(x=w797, y=T13."待机") -> (x != y?=w796:bool)
        n473 = And(x=w780, y=w796) -> (x .and. y?=w781:bool)
        n474 = Select(t="", s=w781, f=w777) -> (s? t:f=w794:string)
        n475 = Select(t="流程结束" ("State(s) In (\"\")"), s=w786, f=w794) -> (s? t:f=w792:string)
        n476 = call "Add State to Queue.vi"("State(s) In Front (\"\")"=w792, "State(s) In (\"\")"=w800) -> ("States Out"=w799:string)  [unwired: 13 in]
      }
      frame "判断质控单元排液是否启动成功" {
        n477 = case shown="真" w823 {
          tunnel: w817 -> [_ w841]
          tunnel: w824 -> [_ w840]
          frame False {
          }
          frame True {
            n478 = call "启动日志.vi"("日志信息"=w841, "Slave ID"=w840) -> ()  [unwired: 9 in, 1 out]
          }
        }
        n479 = case shown="\"CODCr\"" w824 {
          tunnel: [T13."异常停机" ("运行状态") w845 w847 w849 w851 w853] -> w836
          frame "null", Default {
          }
          frame "氨氮" {
            n480 = global read "ZK非断电保存全局变量.vi" "氨氮质控仪器状态"() -> (w846:T18)
            n481 = Unbundle By Name(w846) -> ("运行状态"=w845:T13)
          }
          frame "总磷" {
            n482 = global read "ZK非断电保存全局变量.vi" "总磷质控仪器状态"() -> (w848:T18)
            n483 = Unbundle By Name(w848) -> ("运行状态"=w847:T13)
          }
          frame "总氮" {
            n484 = global read "ZK非断电保存全局变量.vi" "总氮质控仪器状态"() -> (w850:T18)
            n485 = Unbundle By Name(w850) -> ("运行状态"=w849:T13)
          }
          frame "CODMn" {
            n486 = global read "ZK非断电保存全局变量.vi" "CODMn质控仪器状态"() -> (w852:T18)
            n487 = Unbundle By Name(w852) -> ("运行状态"=w851:T13)
          }
          frame "CODCr" {
            n488 = global read "ZK非断电保存全局变量.vi" "CODCr质控仪器状态"() -> (w854:T18)
            n489 = Unbundle By Name(w854) -> ("运行状态"=w853:T13)
          }
        }
        n490 = Index Array(array=w829, index=4 ("索引")) -> (element=w828:refnum<vi>)
        n491 = Greater Or Equal?(x=w822, y=10) -> (x >= y?=w819:bool)
        n492 = property class="DigNum (严格)"(reference=w828) -> ("Value"=w827:u16)  [unwired: 1 in, 2 out]
        n493 = Select(t="质控单元启动排液\n判断质控单元排液是否启动成功" ("State(s) In (\"\")"), s=w819, f=w817) -> (s? t:f=w816:string)
        n494 = Greater Or Equal?(x=w827, y=u16 5) -> (x >= y?=w825:bool)
        n495 = case shown="真" w825 {
          tunnel: w824 -> [_ w843]
          frame False {
          }
          frame True {
            w842 = "质控单元排液启动失败" ("日志信息")
            n496 = call "启动日志.vi"("日志信息"=w842, "Slave ID"=w843) -> ()  [unwired: 9 in, 1 out]
            n497 = call "报警信息记录.vi"("报警信息"=w842, "Slave ID"=w843) -> ()  [unwired: 9 in, 1 out]
          }
        }
        n498 = Not Equal?(x=w836, y=T13."待机") -> (x != y?=w835:bool)
        n499 = And(x=w819, y=w835) -> (x .and. y?=w820:bool)
        n500 = Select(t="", s=w820, f=w816) -> (s? t:f=w833:string)
        n501 = Select(t="流程结束" ("State(s) In (\"\")"), s=w825, f=w833) -> (s? t:f=w831:string)
        n502 = call "Add State to Queue.vi"("State(s) In Front (\"\")"=w831, "State(s) In (\"\")"=w839) -> ("States Out"=w838:string)  [unwired: 13 in]
      }
      frame "质控单元采样中", "质控单元加标中", "质控单元润洗中" {
        n503 = case shown="真" w859 {
          tunnel: w860 -> [_ w879]
          tunnel: w866 -> [_ w878]
          frame False {
          }
          frame True {
            n504 = call "启动日志.vi"("日志信息"=w878, "Slave ID"=w879) -> ()  [unwired: 9 in, 1 out]
          }
        }
        n505 = case shown="\"CODCr\"" w860 {
          tunnel: [T13."待机" ("运行状态") w881 w883 w885 w887 w889] -> w865
          frame "null", Default {
          }
          frame "氨氮" {
            n506 = global read "ZK非断电保存全局变量.vi" "氨氮质控仪器状态"() -> (w882:T18)
            n507 = Unbundle By Name(w882) -> ("运行状态"=w881:T13)
          }
          frame "总磷" {
            n508 = global read "ZK非断电保存全局变量.vi" "总磷质控仪器状态"() -> (w884:T18)
            n509 = Unbundle By Name(w884) -> ("运行状态"=w883:T13)
          }
          frame "总氮" {
            n510 = global read "ZK非断电保存全局变量.vi" "总氮质控仪器状态"() -> (w886:T18)
            n511 = Unbundle By Name(w886) -> ("运行状态"=w885:T13)
          }
          frame "CODMn" {
            n512 = global read "ZK非断电保存全局变量.vi" "CODMn质控仪器状态"() -> (w888:T18)
            n513 = Unbundle By Name(w888) -> ("运行状态"=w887:T13)
          }
          frame "CODCr" {
            n514 = global read "ZK非断电保存全局变量.vi" "CODCr质控仪器状态"() -> (w890:T18)
            n515 = Unbundle By Name(w890) -> ("运行状态"=w889:T13)
          }
        }
        n516 = Greater Or Equal?(x=w858, y=15) -> (x >= y?=w855:bool)
        n517 = Equal?(x=w865, y=T13."异常停机") -> (x = y?=w862:bool)
        n518 = Equal?(x=w865, y=T13."待机") -> (x = y?=w863:bool)
        n519 = Equal?(x=w865, y=T13."等待取样") -> (x = y?=w871:bool)
        n520 = Or(x=w862, y=w863) -> (x .or. y?=w861:bool)
        n521 = And(x=w855, y=w871) -> (x .and. y?=w856:bool)
        n522 = case shown="真" w861 {
          tunnel: w860 -> [_ w877]
          frame False {
          }
          frame True {
            w876 = "质控单元流程中断" ("日志信息")
            n523 = call "启动日志.vi"("日志信息"=w876, "Slave ID"=w877) -> ()  [unwired: 9 in, 1 out]
            n524 = call "报警信息记录.vi"("报警信息"=w876, "Slave ID"=w877) -> ()  [unwired: 9 in, 1 out]
          }
        }
        n525 = Select(t="", s=w856, f=w866) -> (s? t:f=w869:string)
        n526 = Select(t="流程结束" ("State(s) In (\"\")"), s=w861, f=w869) -> (s? t:f=w867:string)
        n527 = call "Add State to Queue.vi"("State(s) In Front (\"\")"=w867, "State(s) In (\"\")"=w875) -> ("States Out"=w874:string)  [unwired: 13 in]
      }
      frame "质控单元排液中" {
        n528 = case shown="真" w895 {
          tunnel: w896 -> [_ w912]
          tunnel: w898 -> [_ w911]
          frame False {
          }
          frame True {
            n529 = call "启动日志.vi"("日志信息"=w911, "Slave ID"=w912) -> ()  [unwired: 9 in, 1 out]
          }
        }
        n530 = case shown="\"CODCr\"" w896 {
          tunnel: [T13."异常停机" ("运行状态") w914 w916 w918 w920 w922] -> w905
          frame "null", Default {
          }
          frame "氨氮" {
            n531 = global read "ZK非断电保存全局变量.vi" "氨氮质控仪器状态"() -> (w915:T18)
            n532 = Unbundle By Name(w915) -> ("运行状态"=w914:T13)
          }
          frame "总磷" {
            n533 = global read "ZK非断电保存全局变量.vi" "总磷质控仪器状态"() -> (w917:T18)
            n534 = Unbundle By Name(w917) -> ("运行状态"=w916:T13)
          }
          frame "总氮" {
            n535 = global read "ZK非断电保存全局变量.vi" "总氮质控仪器状态"() -> (w919:T18)
            n536 = Unbundle By Name(w919) -> ("运行状态"=w918:T13)
          }
          frame "CODMn" {
            n537 = global read "ZK非断电保存全局变量.vi" "CODMn质控仪器状态"() -> (w921:T18)
            n538 = Unbundle By Name(w921) -> ("运行状态"=w920:T13)
          }
          frame "CODCr" {
            n539 = global read "ZK非断电保存全局变量.vi" "CODCr质控仪器状态"() -> (w923:T18)
            n540 = Unbundle By Name(w923) -> ("运行状态"=w922:T13)
          }
        }
        n541 = Greater Or Equal?(x=w894, y=10) -> (x >= y?=w891:bool)
        n542 = Equal?(x=w905, y=T13."异常停机") -> (x = y?=w897:bool)
        n543 = Equal?(x=w905, y=T13."待机") -> (x = y?=w903:bool)
        n544 = And(x=w891, y=w903) -> (x .and. y?=w892:bool)
        n545 = case shown="真" w897 {
          tunnel: w896 -> [_ w910]
          frame False {
          }
          frame True {
            w909 = "质控单元排液流程中断" ("日志信息")
            n546 = call "启动日志.vi"("日志信息"=w909, "Slave ID"=w910) -> ()  [unwired: 9 in, 1 out]
            n547 = call "报警信息记录.vi"("报警信息"=w909, "Slave ID"=w910) -> ()  [unwired: 9 in, 1 out]
          }
        }
        n548 = Select(t="", s=w892, f=w898) -> (s? t:f=w901:string)
        n549 = Select(t="流程结束" ("State(s) In (\"\")"), s=w897, f=w901) -> (s? t:f=w899:string)
        n550 = call "Add State to Queue.vi"("State(s) In Front (\"\")"=w899, "State(s) In (\"\")"=w908) -> ("States Out"=w907:string)  [unwired: 13 in]
      }
      frame "质控单元搅拌中" {
        n551 = case shown="真" w924 {
          tunnel: w925 -> [_ w938]
          tunnel: w930 -> [_ w937]
          frame False {
          }
          frame True {
            n552 = call "启动日志.vi"("日志信息"=w937, "Slave ID"=w938) -> ()  [unwired: 9 in, 1 out]
          }
        }
        n553 = Greater Or Equal?(x=w928, y=15) -> (x >= y?=w926:bool)
        n554 = case shown="真" w926 {
          tunnel: w925 -> [_ w934]
          frame False {
          }
          frame True {
            n555 = call "ZK组合命令区.vi"("是否启用通讯通知"=FALSE, "组合命令区"=质控组合命令区."停止", "Slave ID"=w934) -> ()  [unwired: 8 in, 1 out]
          }
        }
        n556 = Select(t="", s=w926, f=w930) -> (s? t:f=w929:string)
        n557 = call "Add State to Queue.vi"("State(s) In Front (\"\")"=w929, "State(s) In (\"\")"=w933) -> ("States Out"=w932:string)  [unwired: 13 in]
      }
      frame "-------------------# 仪器测试流程 #-------------------" {
        n558 = call "Add State to Queue.vi"("State(s) In (\"\")"=w941) -> ("States Out"=w940:string)  [unwired: 14 in]
      }
      frame "启动仪器水样测试" {
        n559 = Get Date/Time In Seconds() -> (seconds since 1Jan1904=→"水样测试启动时间":timestamp)
        n560 = call "启动日志.vi"("日志信息"=w945, "Slave ID"=w946) -> ()  [unwired: 9 in, 1 out]
        n561 = case shown="\"总氮\"" w946 {
          tunnel: enum16{"水样测试", "平行样测试", "加标回收", "停止"}."水样测试" ("控制命令") -> [_ w955 w956 w957 w958 w959]
          frame "null", Default {
          }
          frame "氨氮" {
            n562 = call "氨氮启动器.vi"("控制命令"=w955) -> ()  [unwired: 11 in]
          }
          frame "总磷" {
            n563 = call "总磷启动器.vi"("控制命令"=w956) -> ()  [unwired: 11 in]
          }
          frame "总氮" {
            n564 = call "总氮启动器.vi"("控制命令"=w957) -> ()  [unwired: 11 in]
          }
          frame "CODMn" {
            n565 = call "CODmn启动器.vi"("控制命令"=w958) -> ()  [unwired: 11 in]
          }
          frame "CODCr" {
            n566 = call "CODcr启动器.vi"("控制命令"=w959) -> ()  [unwired: 11 in]
          }
        }
        n567 = Index Array(array=w949, index=5 ("索引")) -> (element=w948:refnum<vi>)
        n568 = property class="DigNum (严格)"(reference=w948) -> (reference out=w952:refnum<vi>, "Value"=w951:u16)  [unwired: 1 in, 1 out]
        n569 = Increment(x=w951) -> (x+1=w950:u16)
        n570 = property class="DigNum (严格)"(reference=w952, "Value"=w950) -> ()  [unwired: 1 in, 2 out]
        n571 = call "Add State to Queue.vi"("State(s) In (\"\")"=w954) -> ("States Out"=w953:string)  [unwired: 14 in]
      }
      frame "等待仪器空闲" {
        n572 = case shown="真" w960 {
          tunnel: w963 -> [_ w976]
          tunnel: w962 -> [_ w975]
          frame False {
          }
          frame True {
            n573 = call "启动日志.vi"("日志信息"=w975, "Slave ID"=w976) -> ()  [unwired: 9 in, 1 out]
          }
        }
        n574 = case shown="\"总磷\"" w963 {
          tunnel: w962 -> [_ w968]
          tunnel: [_ w967] -> w961
          frame "null", Default {
          }
          frame "总磷" {
            n575 = global read "系统交互.vi" "总磷总氮类型"() -> (w969:enum16{"单模块", "二合一模块"})
            n576 = case shown="\"二合一模块\"" w969 {
              tunnel: w968 -> [_ w972]
              tunnel: [_ w971] -> w967
              frame "单模块", Default {
              }
              frame "二合一模块" {
                n577 = global read "ZK非断电保存全局变量.vi" "流程运行状态标记位"() -> (w974:T7)
                n578 = Unbundle By Name(w974) -> ("总氮"=w973:bool)
                n579 = Select(t=w972, s=w973, f="") -> (s? t:f=w971:string)
              }
            }
          }
        }
        n580 = call "Add State to Queue.vi"("State(s) In Front (\"\")"=w961, "State(s) In (\"\")"=w966) -> ("States Out"=w965:string)  [unwired: 13 in]
      }
      frame "启动仪器加标回收测试" {
        n581 = Get Date/Time In Seconds() -> (seconds since 1Jan1904=→"加标回收启动时间":timestamp)
        n582 = call "启动日志.vi"("日志信息"=w980, "Slave ID"=w981) -> ()  [unwired: 9 in, 1 out]
        n583 = case shown="\"CODMn\"" w981 {
          tunnel: enum16{"水样测试", "平行样测试", "加标回收", "停止"}."加标回收" ("控制命令") -> [_ w990 w991 w992 w993 w994]
          frame "null", Default {
          }
          frame "氨氮" {
            n584 = call "氨氮启动器.vi"("控制命令"=w990) -> ()  [unwired: 11 in]
          }
          frame "总磷" {
            n585 = call "总磷启动器.vi"("控制命令"=w991) -> ()  [unwired: 11 in]
          }
          frame "总氮" {
            n586 = call "总氮启动器.vi"("控制命令"=w992) -> ()  [unwired: 11 in]
          }
          frame "CODMn" {
            n587 = call "CODmn启动器.vi"("控制命令"=w993) -> ()  [unwired: 11 in]
          }
          frame "CODCr" {
            n588 = call "CODcr启动器.vi"("控制命令"=w994) -> ()  [unwired: 11 in]
          }
        }
        n589 = Index Array(array=w984, index=6 ("索引")) -> (element=w983:refnum<vi>)
        n590 = property class="DigNum (严格)"(reference=w983) -> (reference out=w987:refnum<vi>, "Value"=w986:u16)  [unwired: 1 in, 1 out]
        n591 = Increment(x=w986) -> (x+1=w985:u16)
        n592 = property class="DigNum (严格)"(reference=w987, "Value"=w985) -> ()  [unwired: 1 in, 2 out]
        n593 = call "Add State to Queue.vi"("State(s) In (\"\")"=w989) -> ("States Out"=w988:string)  [unwired: 14 in]
      }
      frame "启动仪器平行样测试" {
        n594 = Get Date/Time In Seconds() -> (seconds since 1Jan1904=→"平行样启动时间":timestamp)
        n595 = call "启动日志.vi"("日志信息"=w998, "Slave ID"=w999) -> ()  [unwired: 9 in, 1 out]
        n596 = case shown="\"总磷\"" w999 {
          tunnel: enum16{"水样测试", "平行样测试", "加标回收", "停止"}."平行样测试" ("控制命令") -> [_ w1008 w1009 w1010 w1011 w1012]
          frame "null", Default {
          }
          frame "氨氮" {
            n597 = call "氨氮启动器.vi"("控制命令"=w1008) -> ()  [unwired: 11 in]
          }
          frame "总磷" {
            n598 = call "总磷启动器.vi"("控制命令"=w1009) -> ()  [unwired: 11 in]
          }
          frame "总氮" {
            n599 = call "总氮启动器.vi"("控制命令"=w1010) -> ()  [unwired: 11 in]
          }
          frame "CODMn" {
            n600 = call "CODmn启动器.vi"("控制命令"=w1011) -> ()  [unwired: 11 in]
          }
          frame "CODCr" {
            n601 = call "CODcr启动器.vi"("控制命令"=w1012) -> ()  [unwired: 11 in]
          }
        }
        n602 = Index Array(array=w1002, index=6 ("索引")) -> (element=w1001:refnum<vi>)
        n603 = property class="DigNum (严格)"(reference=w1001) -> (reference out=w1005:refnum<vi>, "Value"=w1004:u16)  [unwired: 1 in, 1 out]
        n604 = Increment(x=w1004) -> (x+1=w1003:u16)
        n605 = property class="DigNum (严格)"(reference=w1005, "Value"=w1003) -> ()  [unwired: 1 in, 2 out]
        n606 = call "Add State to Queue.vi"("State(s) In (\"\")"=w1007) -> ("States Out"=w1006:string)  [unwired: 14 in]
      }
      frame "exit" {
        n607 = call "启动日志.vi"("日志信息"=w1017, "Slave ID"=w1015) -> ()  [unwired: 9 in, 1 out]
        n608 = flat-sequence {
          tunnel: w1015 -> [w1020]
          frame #0 {
            n609 = global read "ZK非断电保存全局变量.vi" "流程运行状态标记位"() -> (w1021:T7)
            n610 = case shown="\"氨氮\"" w1020 {
              tunnel: w1021 -> [_ w1024 w1025 w1028 w1031 w1034]
              frame "null", Default {
              }
              frame "氨氮" {
                n611 = Bundle By Name(cluster=w1024, "氨氮"=FALSE) -> (w1023:T7)
                n612 = global write "ZK非断电保存全局变量.vi" "流程运行状态标记位"(w1023) -> ()
              }
              frame "总磷" {
                n613 = Bundle By Name(cluster=w1025, "总磷"=FALSE ("氨氮")) -> (w1027:T7)
                n614 = global write "ZK非断电保存全局变量.vi" "流程运行状态标记位"(w1027) -> ()
              }
              frame "总氮" {
                n615 = Bundle By Name(cluster=w1028, "总氮"=FALSE ("氨氮")) -> (w1030:T7)
                n616 = global write "ZK非断电保存全局变量.vi" "流程运行状态标记位"(w1030) -> ()
              }
              frame "CODMn" {
                n617 = Bundle By Name(cluster=w1031, "CODMn"=FALSE ("氨氮")) -> (w1033:T7)
                n618 = global write "ZK非断电保存全局变量.vi" "流程运行状态标记位"(w1033) -> ()
              }
              frame "CODCr" {
                n619 = Bundle By Name(cluster=w1034, "CODCr"=FALSE ("氨氮")) -> (w1036:T7)
                n620 = global write "ZK非断电保存全局变量.vi" "流程运行状态标记位"(w1036) -> ()
              }
            }
          }
          frame #1 {
            n621 = global read "ZK非断电保存全局变量.vi" "流程运行状态标记位"() -> (w1040:T7)
            n622 = Cluster To Array(cluster=w1040) -> (array=w1039:bool[])
            n623 = Boolean Array To Number(Boolean array=w1039) -> (number=w1038:u32)
            n624 = Equal To 0?(x=w1038) -> (x = 0?=w1037:bool)
            n625 = case shown="真" w1037 {
              frame False {
              }
              frame True {
                n626 = call "采配水启动器.vi"("启动/停止命令"=T9."停止") -> ()  [unwired: 10 in, 1 out]
              }
            }
          }
        }
        n627 = case shown="\"CODMn\"" w1015 {
          tunnel: enum16{"水样测试", "平行样测试", "加标回收", "停止"}."停止" ("控制命令") -> [_ w1042 w1043 w1044 w1045 w1046]
          frame "null", Default {
          }
          frame "氨氮" {
            n628 = call "氨氮启动器.vi"("控制命令"=w1042) -> ()  [unwired: 11 in]
          }
          frame "总磷" {
            n629 = call "总磷启动器.vi"("控制命令"=w1043) -> ()  [unwired: 11 in]
          }
          frame "总氮" {
            n630 = call "总氮启动器.vi"("控制命令"=w1044) -> ()  [unwired: 11 in]
          }
          frame "CODMn" {
            n631 = call "CODmn启动器.vi"("控制命令"=w1045) -> ()  [unwired: 11 in]
          }
          frame "CODCr" {
            n632 = call "CODcr启动器.vi"("控制命令"=w1046) -> ()  [unwired: 11 in]
          }
        }
        n633 = call "Add State to Queue.vi"("State(s) In Front (\"\")"="流程结束" ("State(s) In Front (\"\")"), "State(s) In (\"\")"=w1019) -> ("States Out"=w1018:string)  [unwired: 13 in]
      }
      frame "判断仪器水样是否启动成功" {
        n634 = case shown="真" w1052 {
          tunnel: w1056 -> [_ w1072]
          tunnel: w1053 -> [_ w1071]
          frame False {
          }
          frame True {
            n635 = call "启动日志.vi"("日志信息"=w1071, "Slave ID"=w1072) -> ()  [unwired: 9 in, 1 out]
          }
        }
        n636 = case shown="\"CODCr\"" w1056 {
          tunnel: [T14."空闲" ("工作状态") w1077 w1079 w1081 w1083 w1085] -> w1068
          frame "null", Default {
          }
          frame "氨氮" {
            w1076 = u16 3 items=["总磷"=1, "总氮"=2, "氨氮"=3, "CODMn"=21] ("站号")
            n637 = call "获取仪器仪表状态.vi"("站号"=w1076) -> ("工作状态"=w1077:T14)  [unwired: 10 in]
          }
          frame "总磷" {
            w1078 = u16 1 items=["总磷"=1, "总氮"=2, "氨氮"=3, "CODMn"=21] ("站号")
            n638 = call "获取仪器仪表状态.vi"("站号"=w1078) -> ("工作状态"=w1079:T14)  [unwired: 10 in]
          }
          frame "总氮" {
            w1080 = u16 2 items=["总磷"=1, "总氮"=2, "氨氮"=3, "CODMn"=21] ("站号")
            n639 = call "获取仪器仪表状态.vi"("站号"=w1080) -> ("工作状态"=w1081:T14)  [unwired: 10 in]
          }
          frame "CODMn" {
            w1082 = u16 21 items=["总磷"=1, "总氮"=2, "氨氮"=3, "CODMn"=21] ("站号")
            n640 = call "获取仪器仪表状态.vi"("站号"=w1082) -> ("工作状态"=w1083:T14)  [unwired: 10 in]
          }
          frame "CODCr" {
            w1084 = u16 22 items=["总磷"=1, "总氮"=2, "氨氮"=3, "CODMn"=21, "CODcr"=22] ("站号")
            n641 = call "获取仪器仪表状态.vi"("站号"=w1084) -> ("工作状态"=w1085:T14)  [unwired: 10 in]
          }
        }
        n642 = Index Array(array=w1061, index=5 ("索引")) -> (element=w1060:refnum<vi>)
        n643 = Greater Or Equal?(x=w1055, y=60) -> (x >= y?=w1048:bool)
        n644 = property class="DigNum (严格)"(reference=w1060) -> ("Value"=w1059:u16)  [unwired: 1 in, 2 out]
        n645 = Greater Or Equal?(x=w1059, y=u16 5) -> (x >= y?=w1057:bool)
        n646 = Equal?(x=w1068, y=T14."空闲") -> (x = y?=w1049:bool)
        n647 = And(x=w1048, y=w1049) -> (x .and. y?=w1047:bool)
        n648 = case shown="真" w1047 {
          tunnel: w1056 -> [_ w1074]
          frame False {
          }
          frame True {
            w1073 = "水样测试启动失败" ("日志信息")
            n649 = call "启动日志.vi"("日志信息"=w1073, "Slave ID"=w1074) -> ()  [unwired: 9 in, 1 out]
            n650 = call "报警信息记录.vi"("报警信息"=w1073, "Slave ID"=w1074) -> ()  [unwired: 9 in, 1 out]
          }
        }
        n651 = Select(t="启动仪器水样测试\n判断仪器水样是否启动成功" ("State(s) In (\"\")"), s=w1049, f="") -> (s? t:f=w1051:string)
        n652 = Select(t=w1051, s=w1048, f=w1053) -> (s? t:f=w1050:string)
        n653 = Select(t="流程结束" ("State(s) In (\"\")"), s=w1057, f=w1050) -> (s? t:f=w1062:string)
        n654 = call "Add State to Queue.vi"("State(s) In Front (\"\")"=w1062, "State(s) In (\"\")"=w1070) -> ("States Out"=w1069:string)  [unwired: 13 in]
      }
      frame "判断仪器加标是否启动成功" {
        n655 = case shown="真" w1092 {
          tunnel: w1091 -> [_ w1111]
          tunnel: w1095 -> [_ w1110]
          frame False {
          }
          frame True {
            n656 = call "启动日志.vi"("日志信息"=w1111, "Slave ID"=w1110) -> ()  [unwired: 9 in, 1 out]
          }
        }
        n657 = case shown="\"CODCr\"" w1095 {
          tunnel: [T14."空闲" ("工作状态") w1116 w1118 w1120 w1122 w1124] -> w1097
          frame "null", Default {
          }
          frame "氨氮" {
            w1115 = u16 3 items=["总磷"=1, "总氮"=2, "氨氮"=3, "CODMn"=21] ("站号")
            n658 = call "获取仪器仪表状态.vi"("站号"=w1115) -> ("工作状态"=w1116:T14)  [unwired: 10 in]
          }
          frame "总磷" {
            w1117 = u16 1 items=["总磷"=1, "总氮"=2, "氨氮"=3, "CODMn"=21] ("站号")
            n659 = call "获取仪器仪表状态.vi"("站号"=w1117) -> ("工作状态"=w1118:T14)  [unwired: 10 in]
          }
          frame "总氮" {
            w1119 = u16 2 items=["总磷"=1, "总氮"=2, "氨氮"=3, "CODMn"=21] ("站号")
            n660 = call "获取仪器仪表状态.vi"("站号"=w1119) -> ("工作状态"=w1120:T14)  [unwired: 10 in]
          }
          frame "CODMn" {
            w1121 = u16 21 items=["总磷"=1, "总氮"=2, "氨氮"=3, "CODMn"=21] ("站号")
            n661 = call "获取仪器仪表状态.vi"("站号"=w1121) -> ("工作状态"=w1122:T14)  [unwired: 10 in]
          }
          frame "CODCr" {
            w1123 = u16 22 items=["总磷"=1, "总氮"=2, "氨氮"=3, "CODMn"=21, "CODcr"=22] ("站号")
            n662 = call "获取仪器仪表状态.vi"("站号"=w1123) -> ("工作状态"=w1124:T14)  [unwired: 10 in]
          }
        }
        n663 = Index Array(array=w1101, index=6 ("索引")) -> (element=w1100:refnum<vi>)
        n664 = Greater Or Equal?(x=w1094, y=60) -> (x >= y?=w1087:bool)
        n665 = property class="DigNum (严格)"(reference=w1100) -> ("Value"=w1099:u16)  [unwired: 1 in, 2 out]
        n666 = Greater Or Equal?(x=w1099, y=u16 5) -> (x >= y?=w1096:bool)
        n667 = Equal?(x=w1097, y=T14."空闲") -> (x = y?=w1088:bool)
        n668 = And(x=w1087, y=w1088) -> (x .and. y?=w1086:bool)
        n669 = case shown="真" w1086 {
          tunnel: w1095 -> [_ w1113]
          frame False {
          }
          frame True {
            w1112 = "加标回收启动失败" ("日志信息")
            n670 = call "启动日志.vi"("日志信息"=w1112, "Slave ID"=w1113) -> ()  [unwired: 9 in, 1 out]
            n671 = call "报警信息记录.vi"("报警信息"=w1112, "Slave ID"=w1113) -> ()  [unwired: 9 in, 1 out]
          }
        }
        n672 = Select(t="启动仪器加标回收测试\n判断仪器加标是否启动成功" ("State(s) In (\"\")"), s=w1088, f="") -> (s? t:f=w1090:string)
        n673 = Select(t=w1090, s=w1087, f=w1091) -> (s? t:f=w1089:string)
        n674 = Select(t="流程结束" ("State(s) In (\"\")"), s=w1096, f=w1089) -> (s? t:f=w1102:string)
        n675 = call "Add State to Queue.vi"("State(s) In Front (\"\")"=w1102, "State(s) In (\"\")"=w1109) -> ("States Out"=w1108:string)  [unwired: 13 in]
      }
      frame "判断仪器平行样是否启动成功" {
        n676 = case shown="真" w1130 {
          tunnel: w1134 -> [_ w1150]
          tunnel: w1131 -> [_ w1149]
          frame False {
          }
          frame True {
            n677 = call "启动日志.vi"("日志信息"=w1149, "Slave ID"=w1150) -> ()  [unwired: 9 in, 1 out]
          }
        }
        n678 = case shown="\"CODCr\"" w1134 {
          tunnel: [T14."空闲" ("工作状态") w1155 w1157 w1159 w1161 w1163] -> w1136
          frame "null", Default {
          }
          frame "氨氮" {
            w1154 = u16 3 items=["总磷"=1, "总氮"=2, "氨氮"=3, "CODMn"=21] ("站号")
            n679 = call "获取仪器仪表状态.vi"("站号"=w1154) -> ("工作状态"=w1155:T14)  [unwired: 10 in]
          }
          frame "总磷" {
            w1156 = u16 1 items=["总磷"=1, "总氮"=2, "氨氮"=3, "CODMn"=21] ("站号")
            n680 = call "获取仪器仪表状态.vi"("站号"=w1156) -> ("工作状态"=w1157:T14)  [unwired: 10 in]
          }
          frame "总氮" {
            w1158 = u16 2 items=["总磷"=1, "总氮"=2, "氨氮"=3, "CODMn"=21] ("站号")
            n681 = call "获取仪器仪表状态.vi"("站号"=w1158) -> ("工作状态"=w1159:T14)  [unwired: 10 in]
          }
          frame "CODMn" {
            w1160 = u16 21 items=["总磷"=1, "总氮"=2, "氨氮"=3, "CODMn"=21] ("站号")
            n682 = call "获取仪器仪表状态.vi"("站号"=w1160) -> ("工作状态"=w1161:T14)  [unwired: 10 in]
          }
          frame "CODCr" {
            w1162 = u16 22 items=["总磷"=1, "总氮"=2, "氨氮"=3, "CODMn"=21, "CODcr"=22] ("站号")
            n683 = call "获取仪器仪表状态.vi"("站号"=w1162) -> ("工作状态"=w1163:T14)  [unwired: 10 in]
          }
        }
        n684 = Index Array(array=w1140, index=6 ("索引")) -> (element=w1139:refnum<vi>)
        n685 = Greater Or Equal?(x=w1133, y=60) -> (x >= y?=w1126:bool)
        n686 = property class="DigNum (严格)"(reference=w1139) -> ("Value"=w1138:u16)  [unwired: 1 in, 2 out]
        n687 = Greater Or Equal?(x=w1138, y=u16 5) -> (x >= y?=w1135:bool)
        n688 = Equal?(x=w1136, y=T14."空闲") -> (x = y?=w1127:bool)
        n689 = And(x=w1126, y=w1127) -> (x .and. y?=w1125:bool)
        n690 = case shown="真" w1125 {
          tunnel: w1134 -> [_ w1152]
          frame False {
          }
          frame True {
            w1151 = "平行样启动失败" ("日志信息")
            n691 = call "启动日志.vi"("日志信息"=w1151, "Slave ID"=w1152) -> ()  [unwired: 9 in, 1 out]
            n692 = call "报警信息记录.vi"("报警信息"=w1151, "Slave ID"=w1152) -> ()  [unwired: 9 in, 1 out]
          }
        }
        n693 = Select(t="启动仪器平行样测试\n判断仪器平行样是否启动成功" ("State(s) In (\"\")"), s=w1127, f="") -> (s? t:f=w1129:string)
        n694 = Select(t=w1129, s=w1126, f=w1131) -> (s? t:f=w1128:string)
        n695 = Select(t="流程结束" ("State(s) In (\"\")"), s=w1135, f=w1128) -> (s? t:f=w1141:string)
        n696 = call "Add State to Queue.vi"("State(s) In Front (\"\")"=w1141, "State(s) In (\"\")"=w1148) -> ("States Out"=w1147:string)  [unwired: 13 in]
      }
      frame "仪器加标回收测试中", "仪器平行样测试中", "仪器水样测试中" {
        n697 = case shown="真" w1168 {
          tunnel: w1170 -> [_ w1190]
          tunnel: w1171 -> [_ w1189]
          frame False {
          }
          frame True {
            n698 = call "启动日志.vi"("日志信息"=w1189, "Slave ID"=w1190) -> ()  [unwired: 9 in, 1 out]
          }
        }
        n699 = case shown="\"CODCr\"" w1170 {
          tunnel: [T14."空闲" ("工作状态") w1180 w1182 w1184 w1186 w1188] -> w1169
          frame "null", Default {
          }
          frame "氨氮" {
            w1179 = u16 3 items=["总磷"=1, "总氮"=2, "氨氮"=3, "CODMn"=21] ("站号")
            n700 = call "获取仪器仪表状态.vi"("站号"=w1179) -> ("工作状态"=w1180:T14)  [unwired: 10 in]
          }
          frame "总磷" {
            w1181 = u16 1 items=["总磷"=1, "总氮"=2, "氨氮"=3, "CODMn"=21] ("站号")
            n701 = call "获取仪器仪表状态.vi"("站号"=w1181) -> ("工作状态"=w1182:T14)  [unwired: 10 in]
          }
          frame "总氮" {
            w1183 = u16 2 items=["总磷"=1, "总氮"=2, "氨氮"=3, "CODMn"=21] ("站号")
            n702 = call "获取仪器仪表状态.vi"("站号"=w1183) -> ("工作状态"=w1184:T14)  [unwired: 10 in]
          }
          frame "CODMn" {
            w1185 = u16 21 items=["总磷"=1, "总氮"=2, "氨氮"=3, "CODMn"=21] ("站号")
            n703 = call "获取仪器仪表状态.vi"("站号"=w1185) -> ("工作状态"=w1186:T14)  [unwired: 10 in]
          }
          frame "CODCr" {
            w1187 = u16 22 items=["总磷"=1, "总氮"=2, "氨氮"=3, "CODMn"=21, "CODcr"=22] ("站号")
            n704 = call "获取仪器仪表状态.vi"("站号"=w1187) -> ("工作状态"=w1188:T14)  [unwired: 10 in]
          }
        }
        n705 = Greater Or Equal?(x=w1167, y=30) -> (x >= y?=w1164:bool)
        n706 = Equal?(x=w1169, y=T14."空闲") -> (x = y?=w1174:bool)
        n707 = And(x=w1164, y=w1174) -> (x .and. y?=w1165:bool)
        n708 = Select(t="", s=w1165, f=w1171) -> (s? t:f=w1172:string)
        n709 = call "Add State to Queue.vi"("State(s) In Front (\"\")"=w1172, "State(s) In (\"\")"=w1177) -> ("States Out"=w1176:string)  [unwired: 13 in]
      }
    }
  }
